vi "mainGUI.vi"() -> ()   [LabVIEW 2025]
uses:
  Photometrics/TPM-LabVIEWSamples/TPM LabVIEW adapter/Camera/Camera.lvclass
  Photometrics/TPM-LabVIEWSamples/TPM LabVIEW adapter/PVCAM/PVCAM.lvclass
  <userlib>/HOLOEYE SLM Display SDK 4.1.0/types/heds_slm_id_typedef.ctl
  <userlib>/HOLOEYE SLM Display SDK 4.1.0/types/heds_required_sdk_version_typedef.ctl
  <vilib>/Utility/error.llb/DialogType.ctl
  channel parameters cluster.ctl
  91398830-3a1b-4311-ae4e-d8b360d25ea5.vi
  <vilib>/DAQmx/write.llb/DAQmx Write (Analog DBL 1Chan 1Samp).vi
  <vilib>/DAQmx/write.llb/DAQmx Write (Analog Wfm 1Chan NSamp).vi
  <vilib>/DAQmx/write.llb/DAQmx Write (Analog 1D Wfm NChan NSamp).vi
  <vilib>/DAQmx/read.llb/DAQmx Read (Analog Wfm 1Chan NSamp).vi
  <vilib>/DAQmx/read.llb/DAQmx Read (Counter U32 1Chan 1Samp).vi
  <vilib>/DAQmx/write.llb/DAQmx Write (Analog 1D DBL NChan 1Samp).vi
  91398830-3a1b-4311-ae4e-d8b360d25ea5.vi/92577ae1-9a41-469a-bc80-42ec99e0da98.vi
  91398830-3a1b-4311-ae4e-d8b360d25ea5.vi/9add13f1-1b17-4127-a253-25fc8ec9b328.vi
  <userlib>/HOLOEYE SLM Display SDK 4.1.0/types/create_heds_data_flags_value.vi
  <userlib>/HOLOEYE SLM Display SDK 4.1.0/misc/heds_sdk_path_v4.1.vi
  <vilib>/Utility/Data Type/Get Type Information.vi
  <vilib>/Utility/Data Type/Get Cluster Information.vi
  <userlib>/HOLOEYE SLM Display SDK 4.1.0/misc/heds_check_error.vi
  <vilib>/DAQmx/miscellaneous.llb/DAQmx Fill In Error Info.vi
  <vilib>/DAQmx/create/channels.llb/DAQmx Create Channel (CI-Count Edges).vi
  <vilib>/DAQmx/create/channels.llb/DAQmx Create Channel (AO-Voltage-Basic).vi
  <vilib>/DAQmx/configure/trigger.llb/DAQmx Start Trigger (Digital Edge).vi
  <resource>/objmgr/daqmx.rc
  <vilib>/Analysis/NI_AALPro.lvlib
  <vilib>/vision/NI_Vision_Development_Module.lvlib
panel:
  in  "Dichroic/dual imaging":bool
  out "SLM image":picture
  out "Kinetix image":picture
  out "594 changed":bool=TRUE
  out "488 changed":bool=TRUE
  out "SLM ID":T1
  in  "Connect SLM":bool
  out "SLM connected":bool
  in  "488 nm LED control":dbl(slide) step=1.0 scale=0.0..100.0 scale format="%#_3g"
  out "Zelux image":picture
  in  "slow camera frequency":u16(ring)=10 caption="Hz" items=["10"=10, "20"=20, "50"=50]
  in  "File prefix":string
  out "488  nm voltage":dbl
  out "594 nm voltage":dbl
  in  "Connect Zelux":bool caption="Connect Kinetix"
  in  "Pulse Duty Cycle":dbl=50.0 caption="%" min=0.0 max=100.0 step=0.1
  in  "Pulse 488":bool
  in  "594 nm laser control":dbl(slide) step=1.0 scale=0.0..100.0 scale format="%#_3g"
  out "PVCam error out":errorcluster
  out "PVCAM Out":refnum<class "PVCAM.lvclass">
  out "Camera obj":refnum<class "Camera.lvclass">
  in  "Connect Kinetix":bool
  in  "Run time":i32 caption="s" min=0
  in  "Begin Experiment":bool
  in  "SLM high":bool
  in  "Load SLM image":bool
  in  "Create SLM image":bool
  in  "Save directory":path=path "D:/KinetixTest/SS_test"
  in  "# Trials":u32=1 caption="trials" min=1 step=1
  in  "Trial Time":dbl=0.1 caption="s" min=0.1 max=60.0 format="%#_2g"
  in  "Run Live":bool caption="Run live"
  in  "scan/fast camera frequency":u16(ring)=100 caption="Hz" items=["20"=20, "100"=100, "800"=800]
  in  "Galvo voltage":dbl=1.0 caption="V" min=0.1 max=1.8 format="%#_2g"
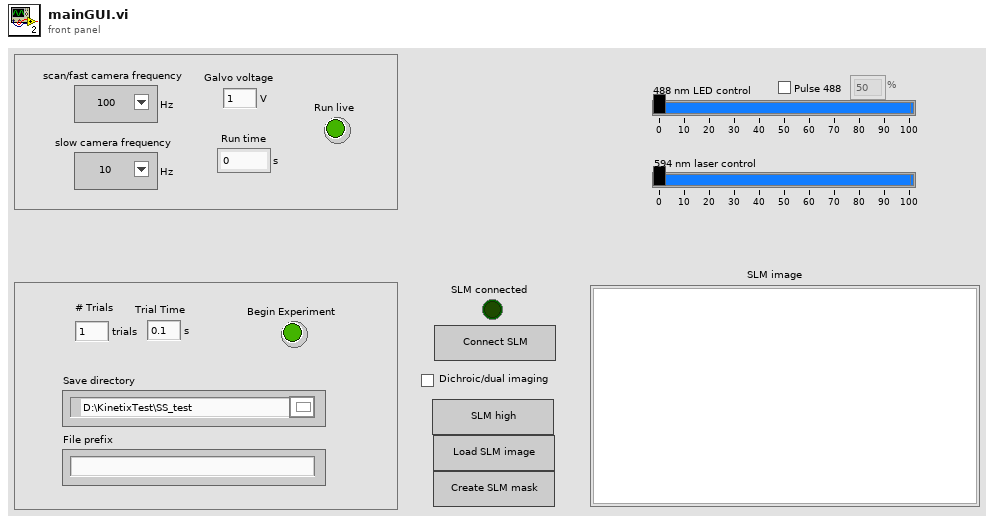
[diagram p1: front panel]
types:
  T1 = typedef "heds_slm_id_typedef.ctl" = cluster{"slmwindow_id":u32, "slmscreen_id":u32}
  T2 = typedef "IMAQ Image.ctl" = refnum<image>
  T3 = typedef "Image Type" = u32
  T4 = typedef "imagedata.ctl" = cluster{"image type":i32, "image depth":i32, "image":u8[], "mask":u8[], "colors":u32[], "Rectangle":cluster{"left":i16, "top":i16, "right":i16, "bottom":i16}}
  T5 = typedef "heds_required_sdk_version_typedef.ctl" = cluster{"Major Version Number":i32, "Minor Version Number":i32}
  T6 = enum8{"Enabled", "Disabled", "Disabled and Grayed Out"}
  T7 = enum16{"open", "open or create", "create or replace", "create", "open (read-only)"}
  T8 = typedef "DialogType.ctl" = u16
  T9 = cluster{"shutter trigger":refnum<k21>, "galvo control":refnum<k21>, "Kinetix trigger":refnum<k21>, "Kinetix readout":refnum<k21>, "Zelux trigger":refnum<k21>, "Zelux readout":refnum<k21>}
  T10 = typedef "channel parameters cluster.ctl" = cluster{"voltage":dbl, "frequency":dbl, "duty cycle":dbl, "sample rate":dbl}
  T11 = cluster{"maximum value":dbl, "minimum value":dbl}
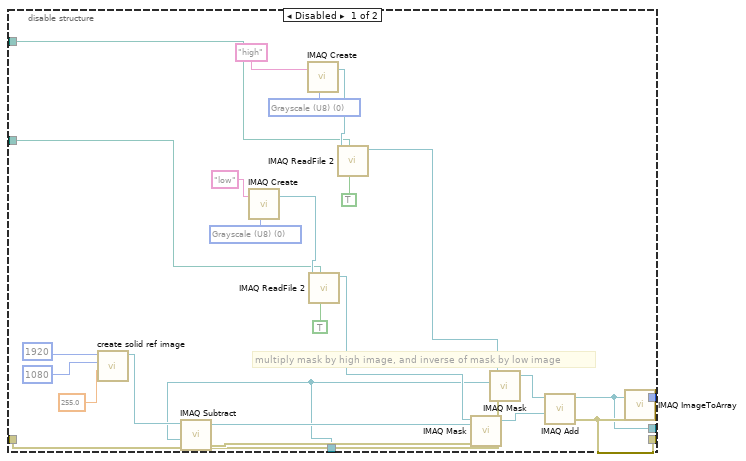
[diagram p3: hidden frame]
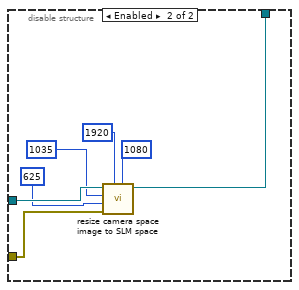
[diagram p4: hidden frame]
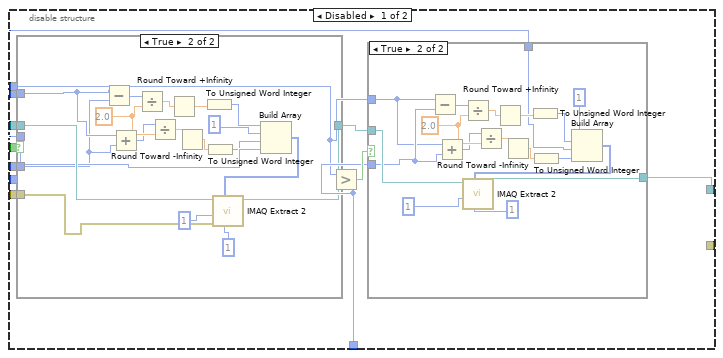
[diagram p5: hidden frame]
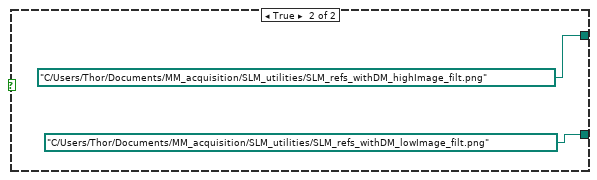
[diagram p8: hidden frame]
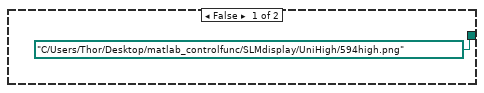
[diagram p10: hidden frame]
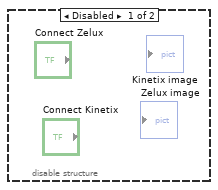
[diagram p14: hidden frame]
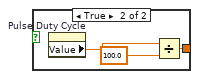
[diagram p17: hidden frame]
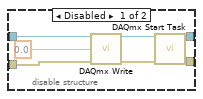
[diagram p18: hidden frame]
diagram:
  # "camera\nopen each in a different window? \n- shows live image\n- allows color scaling\n- allows application of ROI (default and custom)\n\n\n- during run, saves each frame"
  # "todo: \n\n** must stretch masks to fit SLM image\n- resize image based on SLM to camera conversion\n- add zero border to ROI mask if it is too small (assume correct center)\n- crop image if too large (assume correct center)\n\nMake main window not freeze after using slider\n\nstart ThorCam\n\nuse Kinetix without crashing program\n\ndisplay Kinetix and Thorcam during live\n\nin experiment, display and acquire both cameras \n- Kinetix by trial\n-Thorcam throughout\n\n\n\ncheck triggering from BPod (vs function generator - may need to change detection width etc)\n\n\nerror--checking\n- do not fail experiment if 1 camera fails \n\nnon-urgent: \nmake more elegant solution to finish final trial (currently using elapsed time)\nlog BPod trigger in (this is contained in Kinetix data, but can be separated for redundancy)\nadd timeouts for triggers\n\nsave metadata about experiment\n- start time\n- laser and LED power, pulse settings\n- SLM file used (if targeted)\n\nmake parameters file for hardcoded values\n \n\nsave timed experiment and metadata?"
  # "* should calibrate SLM *"
  n1 = case shown="True" "Create SLM image" {
    frame False {
    }
    frame True {
      n2 = flat-sequence {
        tunnel: [w39] -> w35
        tunnel: [w40] -> w34
        tunnel: [w59] -> w38
        tunnel: [w53] -> w37
        tunnel: [w52] -> w36
        tunnel: w35 -> [w46]
        tunnel: w34 -> [w49]
        tunnel: w38 -> [w197]
        tunnel: w37 -> [w196]
        tunnel: w36 -> [w195]
        frame #0 {
          n3 = local read "Save directory"() -> (w43:path)
          n4 = call "IMAQ Load Image Dialog"("Pattern"="*.tif*" ("pattern (all files)"), "Multiple Files? (No)"=FALSE, "Start Path"=w43) -> ("Path"=w42:path)  [unwired: 6 in, 2 out]
          n5 = call "create ROIs GUI.vi"("Mask high value (default 255)"=sgl 255.0, "TIFF path"=w42) -> ("error out"=w40:errorcluster, "ROI mask image"=w39:T2)  [unwired: 8 in]
        }
        frame #1 {
          w51 = 1035 ("y")
          # "if image is correct size or smaller: keep size\nassume center is the same\n\nif image is too large\n\nfinally, resize from image space to SLM space before multiplying with SLM reference images"
          n6 = local read "Dichroic/dual imaging"() -> (w62:bool)
          n7 = case shown="False" w62 {
            tunnel: [path "C:/Users/Thor/Desktop/matlab_controlfunc/SLMdisplay/UniHigh/594high.png" ("path to PNG file") path "C:/Users/Thor/Documents/MM_acquisition/SLM_utilities/SLM_refs_withDM_highImage_filt.png" ("path to PNG file")] -> w61
            tunnel: [path "C:/Users/Thor/Desktop/matlab_controlfunc/SLMdisplay/UniLow/594low.png" ("path to PNG file") path "C:/Users/Thor/Documents/MM_acquisition/SLM_utilities/SLM_refs_withDM_lowImage_filt.png" ("path to PNG file")] -> w60
            frame False {
            }
            frame True {
            }
          }
          n8 = call "IMAQ GetImageInfo"("Image"=w46) -> ("error out"=w57:errorcluster, "Y Resolution"=w54:i32, "X Resolution"=w56:i32)  [unwired: 3 in, 5 out]
          n9 = Greater?(x=w56, y=w51) -> (0:w58:bool)
          n10 = disable-structure shown="Enabled" {
            disable-tunnel: w58 -> [w133 _]
            disable-tunnel: w46 -> [w131 w178]
            disable-tunnel: w57 -> [w129 w175]
            disable-tunnel: w51 -> [w128 _]
            disable-tunnel: w56 -> [w127 w177]
            disable-tunnel: 625 ("y") -> [w126 w180]
            disable-tunnel: w54 -> [w125 w176]
            disable-tunnel: [w124 w173] -> w47
            disable-tunnel: w51 -> [_ w179]
            disable-tunnel: [_ w174] -> w50
            frame Disabled {
              n11 = case shown="True" w133 {
                tunnel: w131 -> [w153 w172]
                tunnel: [w153 w168] -> w130
                tunnel: w129 -> [_ w169]
                tunnel: w127 -> [_ w155]
                tunnel: w128 -> [_ w154]
                tunnel: w125 -> [_ w161]
                frame False {
                }
                frame True {
                  w160 = 2.0 ("y")
                  n12 = Subtract(x=w155, y=w154) -> (x-y=w166:i32)
                  n13 = Add(x=w155, y=w154) -> (x+y=w159:i32)
                  n14 = Divide(x=w166, y=w160) -> (x/y=w165:dbl)
                  n15 = Divide(x=w159, y=w160) -> (x/y=w158:dbl)
                  n16 = Round Toward +Infinity(x=w165) -> (ceil(x): smallest int >= x=w163:dbl)
                  n17 = Round Toward -Infinity(1:w158) -> (0:w157:dbl)
                  n18 = To Unsigned Word Integer(number=w163) -> (unsigned 16bit integer=w164:u16)
                  n19 = To Unsigned Word Integer(number=w157) -> (unsigned 16bit integer=w156:u16)
                  n20 = Build Array(w164, u16 1 ("element"), w156, w161) -> (w167:i32[])
                  n21 = call "IMAQ Extract 2"("Y Step Size"=1, "Optional Rectangle"=w167, "error in (no error)"=w169, "X Step Size"=1, "Image Src"=w172) -> ("Image Dst Out"=w168:T2)  [unwired: 5 in, 1 out]
                }
              }
              n22 = Greater?(x=w125, y=w126) -> (0:w132:bool)
              n23 = case shown="True" w132 {
                tunnel: w130 -> [w134 w152]
                tunnel: [w134 w151] -> w124
                tunnel: w127 -> [_ w138]
                tunnel: w126 -> [_ w137]
                tunnel: w125 -> [_ w136]
                frame False {
                }
                frame True {
                  w145 = 2.0 ("y")
                  n24 = Subtract(x=w136, y=w137) -> (x-y=w148:i32)
                  n25 = Add(x=w136, y=w137) -> (x+y=w144:i32)
                  n26 = Divide(x=w148, y=w145) -> (x/y=w147:dbl)
                  n27 = Divide(x=w144, y=w145) -> (x/y=w143:dbl)
                  n28 = Round Toward +Infinity(x=w147) -> (ceil(x): smallest int >= x=w146:dbl)
                  n29 = Round Toward -Infinity(1:w143) -> (0:w142:dbl)
                  n30 = To Unsigned Word Integer(number=w146) -> (unsigned 16bit integer=w141:u16)
                  n31 = To Unsigned Word Integer(number=w142) -> (unsigned 16bit integer=w140:u16)
                  n32 = Build Array(u16 1 ("element"), w141, w138, w140) -> (w135:i32[])
                  n33 = call "IMAQ Extract 2"("Y Step Size"=1, "Optional Rectangle"=w135, "X Step Size"=1, "Image Src"=w152) -> ("Image Dst Out"=w151:T2)  [unwired: 6 in, 1 out]
                }
              }
            }
            frame Enabled {
              n34 = call "crop_image_to_SLM_size.vi"("Y max"=w180, "X max"=w179, "error in (no error)"=w175, "Y size"=w176, "X size"=w177, "Image Src"=w178) -> ("error out"=w174:errorcluster, "Image Dst Out"=w173:T2)  [unwired: 4 in]
            }
          }
          n35 = disable-structure shown="Disabled" {
            disable-tunnel: w47 -> [w114 w123]
            disable-tunnel: [w99 w121] -> w48
            disable-tunnel: w50 -> [w93 w122]
            frame Disabled {
              w103 = 625 ("Y Resolution")
              w112 = 1035 ("X Resolution")
              n36 = call "IMAQ Create"("Image Name"="correctly sized image") -> ("New Image"=w116:T2)  [unwired: 4 in, 1 out]
              n37 = call "IMAQ GetImageInfo"("error in (no error)"=w93, "Image"=w114) -> ("Y Resolution"=w104:i32, "X Resolution"=w113:i32)  [unwired: 2 in, 6 out]
              n38 = Subtract(x=w112, y=w113) -> (x-y=w111:i32)
              n39 = call "IMAQ SetImageSize"("Y Resolution"=w103, "X Resolution"=w112, "Image"=w116) -> ("Image Out"=w115:T2)  [unwired: 2 in, 1 out]
              n40 = Subtract(x=w103, y=w104) -> (x-y=w108:i32)
              n41 = Divide(x=w111, y=2) -> (x/y=w109:dbl)
              n42 = Divide(x=w108, y=2) -> (x/y=w106:dbl)
              n43 = Round Toward -Infinity(1:w109) -> (0:w105:dbl)
              n44 = Round Toward -Infinity(1:w106) -> (0:w102:dbl)
              n45 = To Unsigned Word Integer(number=w105) -> (unsigned 16bit integer=w97:u16)
              n46 = To Unsigned Word Integer(number=w102) -> (unsigned 16bit integer=w96:u16)
              n47 = Build Array(w97, w96) -> (w95:u16[])
              n48 = call "IMAQ ImageToImage 2"("Offset Left/Top"=w95, "Image Src (Small)"=w114, "Image Src (Large)"=w115) -> ("Image Dst Out"=w98:T2)  [unwired: 7 in, 1 out]
              n49 = call "IMAQ Resample"("X Resolution"=1920, "Y Resolution"=1080, "Image Src"=w98) -> ("Image Dst Out"=w99:T2)  [unwired: 7 in, 1 out]
            }
            frame Enabled {
              n50 = call "resize camera space image to SLM space.vi"("Y SLM"=1080, "X SLM"=1920, "error in (no error)"=w122, "Y camera"=625, "X camera"=1035, "original image"=w123) -> ("Resized image"=w121:T2)  [unwired: 4 in, 1 out]
            }
          }
          n51 = disable-structure shown="Enabled" {
            disable-tunnel: w61 -> [w84 w92]
            disable-tunnel: w60 -> [w78 w91]
            disable-tunnel: [w74 w90] -> w59
            disable-tunnel: [w70 _] -> w53
            disable-tunnel: [w69 w89] -> w52
            disable-tunnel: w49 -> [w68 _]
            disable-tunnel: w48 -> [w63 w88]
            frame Disabled {
              w82 = T3 0 items=["Grayscale (U8)", "Grayscale (I16)", "Grayscale (SGL)", "Complex (CSG)", "RGB (U32)", "HSL (U32)", "RGB (U64)", "Grayscale (U16)"] ("Image Type")
              w87 = T3 0 items=["Grayscale (U8)", "Grayscale (I16)", "Grayscale (SGL)", "Complex (CSG)", "RGB (U32)", "HSL (U32)", "RGB (U64)", "Grayscale (U16)"] ("Image Type")
              # "multiply mask by high image, and inverse of mask by low image"
              n52 = call "create solid ref image.vi"("Pixel Value (default 255)"=sgl 255.0, "Y resolution"=1080 ("Y Resolution"), "X resolution"=1920 ("X Resolution")) -> ("solid image"=w67:T2)  [unwired: 7 in, 1 out]
              n53 = call "IMAQ Subtract"("Image Src A"=w67, "Image Src B"=w63, "error in (no error)"=w68) -> ("Image Dst Out"=w72:T2, "error out"=w75:errorcluster)  [unwired: 4 in]
              n54 = call "IMAQ Create"("Image Name"="low", "Image Type"=w82) -> ("New Image"=w81:T2)  [unwired: 3 in, 1 out]
              n55 = call "IMAQ Create"("Image Name"="high", "Image Type"=w87) -> ("New Image"=w86:T2)  [unwired: 3 in, 1 out]
              n56 = call "IMAQ ReadFile 2"("Use File Path Image Type"=TRUE, "File Path"=w78, "Image"=w81) -> ("Image Out"=w77:T2)  [unwired: 4 in, 4 out]
              n57 = call "IMAQ ReadFile 2"("Use File Path Image Type"=TRUE, "File Path"=w84, "Image"=w86) -> ("Image Out"=w76:T2)  [unwired: 4 in, 4 out]
              n58 = call "IMAQ Mask"("error in (no error)"=w75, "Image Mask"=w72, "Image Src"=w77) -> ("Image Dst Out"=w73:T2)  [unwired: 2 in, 1 out]
              n59 = call "IMAQ Mask"("error in (no error)"=w68, "Image Mask"=w63, "Image Src"=w76) -> ("Image Dst Out"=w71:T2)  [unwired: 2 in, 1 out]
              n60 = call "IMAQ Add"("Image Src A"=w71, "Image Src B"=w73) -> ("Image Dst Out"=w69:T2, "error out"=w70:errorcluster)  [unwired: 5 in]
              n61 = call "IMAQ ImageToArray"("error in (no error)"=w70, "Image"=w69) -> ("Image Pixels (U8)"=w74:u8[][])  [unwired: 2 in, 4 out]
            }
            frame Enabled {
              n62 = call "create SLM image from mask.vi"("low image path"=w91, "high image path"=w92, "Mask"=w88) -> ("Image Pixels (U8)"=w90:u8[][], "Final image"=w89:T2)  [unwired: 7 in]
            }
          }
        }
        frame #2 {
          n63 = property on="File prefix" class="Str"() -> ("Value"=w188:string)  [unwired: 2 in, 2 out]
          n64 = Format Date/Time String(time format string (%c)="%Y%m%d_%H%M%S.png") -> (date/time string=w187:string)  [unwired: 2 in]
          n65 = local read "SLM ID"() -> (w200:T1)
          n66 = Concatenate Strings("SLM_pattern_" ("string"), w188, w187) -> (w190:string)
          n67 = call "load_and_display_SLM.vi"("Image Data"=w197, "SLM ID"=w200) -> ("error out"=w198:errorcluster, "2D Picture"=w199:picture)  [unwired: 8 in]
          n68 = String To Path(string=w190) -> (path=w191:path)
          n69 = property on="Save directory" class="Path"() -> ("Value"=w193:path)  [unwired: 2 in, 2 out]
          n70 = Build Path(base path=w193, name or relative path=w191) -> (appended path=w192:path)
          n71 = property on="SLM image" class="Pict"(error in=w198, "Value"=w199) -> ()  [unwired: 1 in, 2 out]
          n72 = call-poly "IMAQ Write File 2"("Use bit depth? (false)"=TRUE, "error in (no error)"=w196, "Image Quality"=u32 1000, "File Path"=w192, "Image"=w195) -> ()  [unwired: 5 in, 2 out]
        }
        frame #3 {
          n73 = call "IMAQ Dispose"("All Images? (No)"=TRUE) -> ()  [unwired: 5 in, 1 out]
        }
      }
    }
  }
  n74 = case shown="True" "SLM high" {
    tunnel: "Dichroic/dual imaging" -> [_ w204]
    frame False {
    }
    frame True {
      n75 = case shown="True" w204 {
        tunnel: [path "C:/Users/Thor/Desktop/matlab_controlfunc/SLMdisplay/UniHigh/594high.png" ("path to PNG file") path "C:/Users/Thor/Documents/MM_acquisition/SLM_utilities/SLM_refs_withDM_highImage_filt.png" ("path to PNG file")] -> w203
        frame False {
        }
        frame True {
        }
      }
      n76 = call <vilib>:"Check if File or Folder Exists.vi"("path"=w203) -> ("file or folder exists?"=w202:bool)  [unwired: 8 in, 2 out]
      n77 = case shown="True" w202 {
        tunnel: w203 -> [_ w210]
        frame False {
        }
        frame True {
          n78 = call "png_file_to_image_array.vi"("dimension size 2"=1920 ("dimension size"), "dimension size 1"=1080 ("dimension size"), "path to PNG file"=w210) -> ("output array"=w207:u8[][])  [unwired: 8 in]
          n79 = local read "SLM ID"() -> (w213:T1)
          n80 = call "load_and_display_SLM.vi"("Image Data"=w207, "SLM ID"=w213) -> ("error out"=w211:errorcluster, "2D Picture"=w212:picture)  [unwired: 8 in]
          n81 = property on="SLM image" class="Pict"(error in=w211, "Value"=w212) -> ()  [unwired: 1 in, 2 out]
        }
      }
    }
  }
  n82 = case shown="True" "Load SLM image" {
    frame False {
    }
    frame True {
      n83 = property on="Save directory" class="Path"() -> ("Value"=w218:path)  [unwired: 2 in, 2 out]
      n84 = call "File Dialog"("start path"=w218, "pattern (all files)"="*.png") -> ("selected path"=w216:path, "exists"=w214:bool, "error out"=w215:errorcluster)  [unwired: 10 in, 1 out]
      n85 = case shown="True" w214 {
        tunnel: w216 -> [_ w230]
        tunnel: w215 -> [_ w229]
        frame False {
        }
        frame True {
          n86 = local read "SLM ID"() -> (w221:T1)
          n87 = call <vilib>:"Read PNG File.vi"("error in (no error)"=w229, "path to PNG file"=w230) -> ("image data"=w228:T4)  [unwired: 7 in, 2 out]
          n88 = Unbundle By Name(w228) -> ("image"=w226:u8[])  [unwired: 5 out]
          n89 = Reshape Array(w226, 1080 ("dimension size"), 1920 ("dimension size")) -> (w222:u8[][])
          n90 = call "heds_slm_show_imagedata.vim"("Image Data"=w222, "SLM ID"=w221) -> ("error out"=w220:errorcluster, "SLM ID out"=w219:T1)  [unwired: 7 in, 1 out]
          n91 = Unbundle By Name(w219) -> ("slmwindow_id"=w223:u32)
          n92 = call <userlib>:"heds_slmwindow_get_image_data.vi"("error in (no error)"=w220, "slmwindow_id"=w223) -> ("2D Picture"=→"SLM image":picture)  [unwired: 6 in, 3 out]
        }
      }
    }
  }
  n93 = case shown="True" "Connect SLM" {
    frame False {
    }
    frame True {
      n94 = call "connect_SLM.vi"("Required SDK version"=T5 {"Major Version Number"=4, "Minor Version Number"=1}) -> ("SLM connected"=w232:bool, "SLM ID"=→"SLM ID":T1)  [unwired: 9 in]
      "SLM connected" <- w232
      n95 = property on="SLM image" class="Pict"("ZoomFactor"=sgl 0.2 ("Zoom Factor")) -> ()  [unwired: 2 in, 2 out]
      n96 = case shown="True" w232 {
        frame False {
        }
        frame True {
          w235 = T6."Enabled" ("Disabled")
          n97 = property on="Create SLM image" class="Bool"("DisabledEnum"=w235) -> ()  [unwired: 2 in, 2 out]
          n98 = property on="SLM high" class="Bool"("DisabledEnum"=w235) -> ()  [unwired: 2 in, 2 out]
          n99 = property on="Load SLM image" class="Bool"("DisabledEnum"=w235) -> ()  [unwired: 2 in, 2 out]
        }
      }
    }
  }
  n100 = Divide(x="594 nm laser control", y=20.0) -> (x/y=→"594 nm voltage":dbl)
  n101 = disable-structure shown="Enabled" {
    frame Disabled {
    }
    frame Enabled {
    }
  }
  n102 = Divide(x="488 nm LED control", y=20.0) -> (x/y=→"488  nm voltage":dbl)
  n103 = Not(x="Pulse 488") -> (.not. x?=w18:bool)
  n104 = Boolean To (0,1)(Boolean=w18) -> (0, 1=w19:i16)
  n105 = Multiply(x=w19, y=2.0) -> (x*y=w20:dbl)
  n106 = property on="Pulse Duty Cycle" class="DigNum (strict)"("DisabledEnum"=w20) -> ()  [unwired: 2 in, 2 out]
  n107 = property on="Begin Experiment" class="Bool (strict)"() -> ("Value"=w10:bool)  [unwired: 2 in, 2 out]
  n108 = property on="Run Live" class="Bool (strict)"() -> ("Value"=w30:bool)  [unwired: 2 in, 2 out]
  n109 = Boolean To (0,1)(Boolean=w30) -> (0, 1=w31:i16)
  n110 = Boolean To (0,1)(Boolean=w10) -> (0, 1=w27:i16)
  n111 = case shown="True" w30 {
    tunnel: ["Run live" "End live"] -> w33
    frame False {
    }
    frame True {
    }
  }
  n112 = case shown="False" w10 {
    tunnel: ["Begin Experiment" "End experiment"] -> w25
    frame False {
    }
    frame True {
    }
  }
  n113 = Multiply(x=w31, y=2.0) -> (x*y=w29:dbl)
  n114 = Multiply(x=w27, y=2.0) -> (x*y=w26:dbl)
  n115 = property on="Begin Experiment" class="Bool (strict)"("DisabledEnum"=w29) -> ()  [unwired: 2 in, 2 out]
  n116 = property on="Run Live" class="Bool (strict)"("DisabledEnum"=w26) -> ()  [unwired: 2 in, 2 out]
  n117 = disable-structure shown="Enabled" {
    disable-tunnel: w10 -> [w245 _]
    disable-tunnel: "Trial Time" -> [w244 _]
    disable-tunnel: "scan/fast camera frequency" -> [w243 _]
    disable-tunnel: "slow camera frequency" -> [w242 _]
    disable-tunnel: "# Trials" -> [w241 _]
    disable-tunnel: "Galvo voltage" -> [w240 _]
    frame Disabled {
      n118 = case shown="True" w245 {
        tunnel: w243 -> [_ w414]
        tunnel: w240 -> [_ w413]
        tunnel: w244 -> [_ w272]
        tunnel: w241 -> [_ w412]
        tunnel: w242 -> [_ w291]
        tunnel: w242 -> [_ w269]
        frame False {
        }
        frame True {
          w307 = T8 0 items=["no dialog", "OK message", "continue or stop message", "OK message + warnings", "continue/stop + warnings"] ("type of dialog (OK msg:1)")
          w313 = 10123 items=["Finite Samples"=10178, "Continuous Samples"=10123, "Hardware Timed Single Point"=12522] ("SampQuant.SampMode")
          w318 = T8 0 items=["no dialog", "OK message", "continue or stop message", "OK message + warnings", "continue/stop + warnings"] ("type of dialog (OK msg:1)")
          w325 = 10123 items=["Finite Samples"=10178, "Continuous Samples"=10123, "Hardware Timed Single Point"=12522] ("SampQuant.SampMode")
          w337 = 10178 items=["Finite Samples"=10178, "Continuous Samples"=10123, "Hardware Timed Single Point"=12522] ("SampQuant.SampMode")
          w278 = 10178 items=["Finite Samples"=10178, "Continuous Samples"=10123, "Hardware Timed Single Point"=12522] ("SampQuant.SampMode")
          w350 = 10123 items=["Finite Samples"=10178, "Continuous Samples"=10123, "Hardware Timed Single Point"=12522] ("SampQuant.SampMode")
          w373 = 10280 items=["Rising"=10280, "Falling"=10171] ("edge")
          w261 = tag "/GalvoPMT/PFI9" ("source")
          w356 = 10178 items=["Finite Samples"=10178, "Continuous Samples"=10123, "Hardware Timed Single Point"=12522] ("SampQuant.SampMode")
          w408 = T8 0 items=["no dialog", "OK message", "continue or stop message", "OK message + warnings", "continue/stop + warnings"] ("type of dialog (OK msg:1)")
          w410 = T8 0 items=["no dialog", "OK message", "continue or stop message", "OK message + warnings", "continue/stop + warnings"] ("type of dialog (OK msg:1)")
          # "min pulse width ensures proper increment/debouncing"
          n119 = call-poly <vilib>:"DAQmx Create Virtual Channel.vi"("maximum value"=5.0, "minimum value"=0.0, "physical channels"=tag "PZT/ao0", "name to assign"="488 nm") -> ("task out"=w289:refnum<k21>, "error out"=w290:errorcluster)  [unwired: 10 in]
          n120 = property class="DAQmx Timing"(reference=w289, error in=w290, "Sample Quantity:Sample Mode"=w325) -> (reference out=w323:refnum<k21>, error out=w322:errorcluster)
          n121 = property on="488  nm voltage" class="DigNum (strict)"() -> ("Value"=w293:dbl)  [unwired: 2 in, 2 out]
          n122 = property on="Pulse 488" class="Bool (strict)"() -> ("Value"=w326:bool)  [unwired: 2 in, 2 out]
          n123 = case shown="True" w326 {
            tunnel: [w416 w425] -> w324
            tunnel: w323 -> [w418 w427]
            tunnel: [w415 w424] -> w321
            tunnel: w322 -> [w419 w428]
            tunnel: w293 -> [w417 w430]
            tunnel: w291 -> [_ w420]
            frame False {
              n124 = call-poly <vilib>:"DAQmx Write.vi"("task/channels in"=w418, "data"=w417, "error in"=w419) -> ("task out"=w416:refnum<k21>, "error out"=w415:errorcluster)  [unwired: 10 in, 1 out]
            }
            frame True {
              # "need to copy loop in free run case (after fixing it)"
              n125 = property on="Pulse Duty Cycle" class="DigNum (strict)"() -> ("Value"=w423:dbl)  [unwired: 2 in, 2 out]
              n126 = property class="DAQmx Timing"(reference=w427) -> ("SampClk.Rate"=w429:dbl)  [unwired: 1 in, 2 out]
              n127 = Divide(x=w423, y=100.0) -> (x/y=w421:dbl)
              n128 = Divide(x=1.0, y=w420) -> (x/y=w431:dbl)
              n129 = call "make step function for duty cycle.vi"("amplitude"=w430, "period"=w431, "duty cycle"=w421, "sample rate"=w429) -> ("Waveform out"=w426:waveform(dbl))  [unwired: 7 in]
              n130 = call-poly <vilib>:"DAQmx Write.vi"("task/channels in"=w427, "data"=w426, "error in"=w428) -> ("task out"=w425:refnum<k21>, "error out"=w424:errorcluster)  [unwired: 10 in, 1 out]
            }
          }
          n131 = call "init_DAQ_cluster.vi"("Sample rate"=100000.0, "Slow/Zelux frame frequency"=w269, "Fast/Kinetix frame frequency"=w414) -> ("error out"=w270:errorcluster, "tasks cluster"=w274:T9)  [unwired: 7 in]
          n132 = Unbundle By Name(w274) -> ("shutter trigger"=w273:refnum<k21>, "galvo control"=w254:refnum<k21>, "Kinetix trigger"=w256:refnum<k21>, "Zelux trigger"=w260:refnum<k21>, "Kinetix readout"=w257:refnum<k21>, "Zelux readout"=w258:refnum<k21>)
          n133 = property class="DAQmx Timing"(reference=w254) -> ("SampClk.Rate"=w338:dbl)  [unwired: 1 in, 2 out]
          n134 = call-poly <vilib>:"DAQmx Trigger.vi"("task/channels in"=w254, "source"=w261, "error in"=w270) -> ("task out"=w405:refnum<k21>, "error out"=w404:errorcluster)  [unwired: 11 in]
          n135 = property on="File prefix" class="Str"() -> ("Value"=w263:string)  [unwired: 2 in, 2 out]
          n136 = property class="DAQmx Channel"(reference=w260, error in=w270) -> ("CO.Pulse.Freq"=w271:dbl)  [unwired: 2 out]
          n137 = property class="DAQmx Channel"(reference=w256, error in=w270) -> ("CO.Pulse.Freq"=w292:dbl)  [unwired: 2 out]
          n138 = property class="DAQmx Timing"(reference=w254) -> ("SampClk.Rate"=w353:dbl)  [unwired: 1 in, 2 out]
          n139 = property class="DAQmx Trigger"(reference=w405, error in=w404, "Start.Retriggerable"=TRUE) -> (reference out=w361:refnum<k21>)  [unwired: 1 out]
          n140 = Concatenate Strings(w263, "_Kinetix.tdms") -> (w268:string)
          n141 = Concatenate Strings(w263, "_Zelux.tdms") -> (w264:string)
          n142 = call-poly <vilib>:"DAQmx Create Virtual Channel.vi"("maximum value"=5.0, "minimum value"=0.0, "physical channels"=tag "PZT/ao1", "name to assign"="594 nm") -> ("task out"=w315:refnum<k21>, "error out"=w314:errorcluster)  [unwired: 10 in]
          n143 = Divide(x=1.0, y=w272) -> (x/y=w370:dbl)
          n144 = Multiply(x=w271, y=w272) -> ()  [unwired: 1 out]
          n145 = property class="DAQmx Channel"(reference=w273, error in=w270, "CO.Pulse.Freq"=w370) -> (reference out=w372:refnum<k21>)  [unwired: 1 out]
          n146 = property on="594 nm voltage" class="DigNum (strict)"() -> ("Value"=w316:dbl)  [unwired: 2 in, 2 out]
          n147 = Multiply(x=w292, y=w272) -> (x*y=w354:dbl)
          n148 = Multiply(x=w353, y=w272) -> (x*y=w355:dbl)
          n149 = String To Path(string=w268) -> (path=w266:path)
          n150 = String To Path(string=w264) -> (path=w265:path)
          n151 = call-poly <vilib>:"DAQmx Trigger.vi"("task/channels in"=w256, "source"=w261) -> ("task out"=w391:refnum<k21>, "error out"=w390:errorcluster)  [unwired: 12 in]
          n152 = call "galvo_triangle_wave.vi"("trial seconds"=w272, "final frequency"=w292, "amplitude"=w413, "sample rate"=w353) -> ("waveform array out"=w367:waveform(dbl)[])  [unwired: 7 in]
          n153 = property class="DAQmx Trigger"(reference=w391, error in=w390, "Start.Retriggerable"=TRUE) -> (reference out=w357:refnum<k21>, error out=w358:errorcluster)
          n154 = call-poly <vilib>:"DAQmx Write.vi"("task/channels in"=w315, "data"=w316, "error in"=w314) -> ("task out"=w312:refnum<k21>, "error out"=w311:errorcluster)  [unwired: 10 in, 1 out]
          n155 = call-poly <vilib>:"DAQmx Create Virtual Channel.vi"("initial count"=u32 0, "edge"=w373, "counter"=tag "GalvoPMT/ctr1") -> ("task out"=w402:refnum<k21>, "error out"=w401:errorcluster)  [unwired: 11 in]
          n156 = call-poly <vilib>:"DAQmx Trigger.vi"("task/channels in"=w372, "source"=w261) -> ("task out"=w388:refnum<k21>, "error out"=w389:errorcluster)  [unwired: 12 in]
          n157 = property on="Save directory" class="Path"() -> ("Value"=w349:path)  [unwired: 2 in, 2 out]
          n158 = property on="Save directory" class="Path"() -> ("Value"=w284:path)  [unwired: 2 in, 2 out]
          n159 = property class="DAQmx Timing"(reference=w361, "Sample Quantity:Sample Mode"=w356, "SampQuant.SampPerChan"=w355) -> (reference out=w362:refnum<k21>)  [unwired: 1 in, 1 out]
          n160 = property class="DAQmx Channel"(reference=w402, error in=w401, "CI.CountEdges.Term"=w261, "CI.CountEdges.DigFltr.MinPulseWidth"=1e-06 ("DI.DigFltr.MinPulseWidth")) -> (reference out=w395:refnum<k21>, error out=w394:errorcluster)
          n161 = property class="DAQmx Trigger"(reference=w388, error in=w389, "Start.Retriggerable"=TRUE) -> (reference out=w387:refnum<k21>)  [unwired: 1 out]
          n162 = Build Path(base path=w349, name or relative path=w266) -> (appended path=w345:path)
          n163 = Build Path(base path=w284, name or relative path=w265) -> (appended path=w283:path)
          n164 = call-poly <vilib>:"DAQmx Trigger.vi"("task/channels in"=w257, "source"=w261) -> ("task out"=w248:refnum<k21>, "error out"=w346:errorcluster)  [unwired: 12 in]
          n165 = call-poly <vilib>:"DAQmx Trigger.vi"("task/channels in"=w258, "source"=w261) -> ("task out"=w251:refnum<k21>, "error out"=w250:errorcluster)  [unwired: 12 in]
          n166 = Multiply(x=w272, y=w338) -> (x*y=w277:dbl)
          n167 = property class="DAQmx Timing"(reference=w357, error in=w358, "Sample Quantity:Sample Mode"=w337, "SampQuant.SampPerChan"=w354) -> (reference out=w360:refnum<k21>, error out=w359:errorcluster)
          n168 = property class="DAQmx Timing"(reference=w248, "Sample Quantity:Sample Mode"=w278, "SampQuant.SampPerChan"=w277) -> (reference out=w247:refnum<k21>)  [unwired: 1 in, 1 out]
          n169 = property class="DAQmx Timing"(reference=w251, error in=w250, "Sample Quantity:Sample Mode"=w278, "SampQuant.SampPerChan"=w277) -> (reference out=w253:refnum<k21>, error out=w249:errorcluster)
          n170 = property class="DAQmx Timing"(reference=w312, error in=w311, "Sample Quantity:Sample Mode"=w313) -> (reference out=w310:refnum<k21>, error out=w309:errorcluster)
          n171 = call-poly <vilib>:"DAQmx Write.vi"("task/channels in"=w362, "data"=w367, "error in"=w270) -> ("task out"=w366:refnum<k21>, "error out"=w365:errorcluster)  [unwired: 10 in, 1 out]
          n172 = property class="DAQmx Trigger"(reference=w247, "Start.Retriggerable"=TRUE) -> (reference out=w259:refnum<k21>)  [unwired: 1 in, 1 out]
          n173 = property class="DAQmx Trigger"(reference=w253, error in=w249, "Start.Retriggerable"=TRUE) -> (reference out=w276:refnum<k21>, error out=w275:errorcluster)
          n174 = call <vilib>:"DAQmx Start Task.vi"("task/channels in"=w360, "error in"=w359) -> ("task out"=w382:refnum<k21>, "error out"=w381:errorcluster)  [unwired: 12 in]
          n175 = call <vilib>:"DAQmx Start Task.vi"("task/channels in"=w395, "error in"=w394) -> ("task out"=w393:refnum<k21>, "error out"=w392:errorcluster)  [unwired: 12 in]
          n176 = call <vilib>:"DAQmx Start Task.vi"("task/channels in"=w310, "error in"=w309) -> ("task out"=w305:refnum<k21>, "error out"=w304:errorcluster)  [unwired: 12 in]
          n177 = call <vilib>:"DAQmx Start Task.vi"("task/channels in"=w366, "error in"=w365) -> ("task out"=w364:refnum<k21>, "error out"=w363:errorcluster)  [unwired: 12 in]
          n178 = call <vilib>:"DAQmx Start Task.vi"("task/channels in"=w387, "error in"=w270) -> ("task out"=w378:refnum<k21>, "error out"=w375:errorcluster)  [unwired: 12 in]
          n179 = TDMS Open(10:T7."open or create" ("operation (0:open)"), 11:w345) -> (0:w342:errorcluster, 3:w344:refnum<k34>)  [unwired: 5 in]
          n180 = TDMS Open(10:T7."open or create" ("operation (0:open)"), 11:w283) -> (0:w279:errorcluster, 3:w282:refnum<k34>)  [unwired: 5 in]
          n181 = call <vilib>:"DAQmx Start Task.vi"("task/channels in"=w324, "error in"=w321) -> ("task out"=w320:refnum<k21>, "error out"=w317:errorcluster)  [unwired: 12 in]
          n182 = while {
            tunnel: w412 -> [w459]
            tunnel: [w483] -> w399
            tunnel: [w482] -> w397
            tunnel: w393 -> [w479]
            tunnel: w392 -> [w478]
            tunnel: [w472] -> w384
            tunnel: [w469] -> w383
            tunnel: w382 -> [w476]
            tunnel: w381 -> [w477]
            tunnel: [w477] -> w380
            tunnel: [w476] -> w379
            tunnel: w378 -> [w468]
            tunnel: [w468] -> w377
            tunnel: [w475] -> w376
            tunnel: w375 -> [w475]
            tunnel: [FALSE] -> w369
            tunnel: w364 -> [w469]
            tunnel: w363 -> [w472]
            tunnel: w272 -> [w467]
            tunnel: w259 -> [w461]
            tunnel: w344 -> [w465]
            tunnel: [w464] -> w343
            tunnel: w342 -> [w466]
            tunnel: [w463] -> w341
            tunnel: [w462] -> w340
            tunnel: w277 -> [_]
            tunnel: [w457] -> w297
            tunnel: w320 -> [w457]
            tunnel: [w456] -> w296
            tunnel: w317 -> [w456]
            tunnel: [w455] -> w306
            tunnel: w305 -> [w455]
            tunnel: w304 -> [w454]
            tunnel: [w454] -> w303
            tunnel: [w453] -> w288
            tunnel: [w452] -> w287
            tunnel: w282 -> [w451]
            tunnel: [w450] -> w280
            tunnel: w279 -> [w449]
            tunnel: w276 -> [w436]
            stop <- w474 stop-if-true
            # "Run experiment"
            n183 = call-poly <vilib>:"DAQmx Read.vi"("task/channels in"=w479, "error in"=w478) -> ("task out"=w483:refnum<k21>, "data"=w481:u32, "error out"=w482:errorcluster)  [unwired: 11 in]
            n184 = call-poly <vilib>:"DAQmx Read.vi"("task/channels in"=w461) -> ("task out"=w462:refnum<k21>, "data"=w434:waveform(dbl))  [unwired: 12 in, 1 out]
            n185 = call-poly <vilib>:"DAQmx Read.vi"("task/channels in"=w436) -> ("task out"=w450:refnum<k21>, "data"=w433:waveform(dbl))  [unwired: 12 in, 1 out]
            n186 = Subtract(x=w459, y=u32 1) -> (x-y=w458:u32)
            n187 = Wait (ms)(milliseconds to wait=u32 10) -> ()  [unwired: 1 out]
            n188 = Greater Or Equal?(x=w481, y=w458) -> (x >= y?=w471:bool)
            n189 = Unbundle By Name(w434) -> ("t0"=w443:timestamp, "dt"=w446:dbl)  [unwired: 1 out]
            n190 = Unbundle By Name(w433) -> ("t0"=w437:timestamp, "dt"=w440:dbl)  [unwired: 1 out]
            n191 = call <vilib>:"Threshold Detector.vi"("threshold"=1.0, "X"=w434) -> ("Indices"=w447:i32[])  [unwired: 1 in, 2 out]
            n192 = call <vilib>:"Threshold Detector.vi"("threshold"=1.0, "X"=w433) -> ("Indices"=w441:i32[])  [unwired: 1 in, 2 out]
            n193 = Multiply(x=w447, y=w446) -> (x*y=w445:dbl[])
            n194 = Multiply(x=w441, y=w440) -> (x*y=w439:dbl[])
            n195 = case shown="True" w471 {
              selector: w471 -> [w485 _]
              tunnel: [w485 w487] -> w470
              tunnel: w467 -> [_ w486]
              frame False {
              }
              frame True {
                n196 = while {
                  tunnel: [w488] -> w487
                  tunnel: w486 -> [w489]
                  stop <- w488 stop-if-true
                  n197 = call "Elapsed Time"("Time Target (s)"=w489) -> ("Time has Elapsed"=w488:bool)  [unwired: 11 in, 7 out]
                }
              }
            }
            n198 = Add(x=w445, y=w443) -> (x+y=w448:timestamp[])
            n199 = Add(x=w439, y=w437) -> (x+y=w442:timestamp[])
            n200 = TDMS Write(0:w465, 9:w448, 11:w466) -> (4:w464:refnum<k34>, 15:w463:errorcluster)  [unwired: 3 in, 2 out]
            n201 = TDMS Write(0:w451, 9:w442, 11:w449) -> (4:w452:refnum<k34>, 15:w453:errorcluster)  [unwired: 3 in, 2 out]
            n202 = property on="Begin Experiment" class="Bool (strict)"() -> ("Value"=w435:bool)  [unwired: 2 in, 2 out]
            n203 = Not(x=w435) -> (.not. x?=w484:bool)
            n204 = Or(x=w470, y=w484) -> (x .or. y?=w474:bool)
          }
          n205 = property on="Begin Experiment" class="Bool (strict)"("Value"=w369) -> ()  [unwired: 2 in, 2 out]
          n206 = TDMS Close(8:w341, 11:w343) -> ()  [unwired: 2 out]
          n207 = TDMS Close(8:w288, 11:w287) -> ()  [unwired: 2 out]
          n208 = call <vilib>:"DAQmx Stop Task.vi"("task/channels in"=w379, "error in"=w380) -> ("task out"=w406:refnum<k21>, "error out"=w407:errorcluster)  [unwired: 12 in]
          n209 = call <vilib>:"DAQmx Stop Task.vi"("task/channels in"=w399, "error in"=w397) -> ("task out"=w398:refnum<k21>, "error out"=w396:errorcluster)  [unwired: 12 in]
          n210 = call <vilib>:"DAQmx Stop Task.vi"("task/channels in"=w297, "error in"=w296) -> ("task out"=w300:refnum<k21>, "error out"=w301:errorcluster)  [unwired: 12 in]
          n211 = call <vilib>:"DAQmx Clear Task.vi"("task in"=w306, "error in"=w303) -> ("error out"=w308:errorcluster)  [unwired: 13 in]
          n212 = call <vilib>:"DAQmx Stop Task.vi"("task/channels in"=w383, "error in"=w384) -> ("task out"=w352:refnum<k21>, "error out"=w351:errorcluster)  [unwired: 12 in]
          n213 = call <vilib>:"DAQmx Clear Task.vi"("task in"=w377, "error in"=w376) -> ("error out"=w409:errorcluster)  [unwired: 13 in]
          n214 = call <vilib>:"DAQmx Stop Task.vi"("task/channels in"=w340, "error in"=w346) -> ("task out"=w348:refnum<k21>, "error out"=w347:errorcluster)  [unwired: 12 in]
          n215 = call <vilib>:"DAQmx Stop Task.vi"("task/channels in"=w280, "error in"=w275) -> ("task out"=w286:refnum<k21>, "error out"=w285:errorcluster)  [unwired: 12 in]
          n216 = call <vilib>:"DAQmx Clear Task.vi"("task in"=w398, "error in"=w396) -> ()  [unwired: 13 in, 1 out]
          n217 = call <vilib>:"DAQmx Clear Task.vi"("task in"=w348, "error in"=w347) -> ()  [unwired: 13 in, 1 out]
          n218 = call <vilib>:"DAQmx Clear Task.vi"("task in"=w286, "error in"=w285) -> ()  [unwired: 13 in, 1 out]
          n219 = call <vilib>:"DAQmx Clear Task.vi"("task in"=w406, "error in"=w407) -> ("error out"=w411:errorcluster)  [unwired: 13 in]
          n220 = call <vilib>:"Simple Error Handler.vi"("type of dialog (OK msg:1)"=w307, "error in (no error)"=w308) -> ()  [unwired: 3 in, 5 out]
          n221 = property class="DAQmx Timing"(reference=w352, error in=w351, "Sample Quantity:Sample Mode"=w350) -> (reference out=w336:refnum<k21>, error out=w335:errorcluster)
          n222 = call <vilib>:"Simple Error Handler.vi"("type of dialog (OK msg:1)"=w408, "error in (no error)"=w409) -> ()  [unwired: 3 in, 5 out]
          n223 = call-poly <vilib>:"DAQmx Write.vi"("task/channels in"=w300, "data"=0.0, "error in"=w301) -> ("task out"=w299:refnum<k21>, "error out"=w298:errorcluster)  [unwired: 10 in, 1 out]
          n224 = call <vilib>:"Simple Error Handler.vi"("type of dialog (OK msg:1)"=w410, "error in (no error)"=w411) -> ()  [unwired: 3 in, 5 out]
          n225 = call <vilib>:"DAQmx Start Task.vi"("task/channels in"=w299, "error in"=w298) -> ("task out"=w295:refnum<k21>, "error out"=w294:errorcluster)  [unwired: 12 in]
          n226 = call "galvo_recenter.vi"("error in"=w335, "task/channels in"=w336) -> ()  [unwired: 10 in]
          n227 = call <vilib>:"DAQmx Clear Task.vi"("task in"=w295, "error in"=w294) -> ("error out"=w319:errorcluster)  [unwired: 13 in]
          n228 = call <vilib>:"Simple Error Handler.vi"("type of dialog (OK msg:1)"=w318, "error in (no error)"=w319) -> ()  [unwired: 3 in, 5 out]
        }
      }
    }
    frame Enabled {
    }
  }
  n229 = disable-structure shown="Enabled" {
    disable-tunnel: w10 -> [w495 _]
    disable-tunnel: "Trial Time" -> [w494 _]
    disable-tunnel: "# Trials" -> [w493 _]
    disable-tunnel: "Galvo voltage" -> [w492 _]
    disable-tunnel: "slow camera frequency" -> [w491 _]
    disable-tunnel: "scan/fast camera frequency" -> [w490 _]
    frame Enabled {
      n230 = case shown="True" w495 {
        tunnel: w490 -> [_ w685]
        tunnel: w492 -> [_ w565]
        tunnel: w494 -> [_ w561]
        tunnel: w493 -> [_ w611]
        tunnel: w491 -> [_ w614]
        frame False {
        }
        frame True {
          w538 = 10123 items=["Finite Samples"=10178, "Continuous Samples"=10123, "Hardware Timed Single Point"=12522] ("SampQuant.SampMode")
          w546 = 10150 items=["Analog Edge"=10099, "Analog Multi Edge"=16108, "Digital Edge"=10150, "Digital Pattern"=10398, "Analog Window"=10103, "Time"=15996, "None"=10230] ("Start.TrigType")
          w557 = 10388 items=["Sample Clock"=10388, "Burst Handshake"=12548, "Handshake"=10389, "Implicit"=10451, "On Demand"=10390, "Change Detection"=12504, "Pipelined Sample Clock"=14668] ("SampTimingType")
          w580 = T8 0 items=["no dialog", "OK message", "continue or stop message", "OK message + warnings", "continue/stop + warnings"] ("type of dialog (OK msg:1)")
          w589 = T8 0 items=["no dialog", "OK message", "continue or stop message", "OK message + warnings", "continue/stop + warnings"] ("type of dialog (OK msg:1)")
          w625 = T8 0 items=["no dialog", "OK message", "continue or stop message", "OK message + warnings", "continue/stop + warnings"] ("type of dialog (OK msg:1)")
          w642 = 10123 items=["Finite Samples"=10178, "Continuous Samples"=10123, "Hardware Timed Single Point"=12522] ("SampQuant.SampMode")
          w645 = T8 0 items=["no dialog", "OK message", "continue or stop message", "OK message + warnings", "continue/stop + warnings"] ("type of dialog (OK msg:1)")
          w648 = 10178 items=["Finite Samples"=10178, "Continuous Samples"=10123, "Hardware Timed Single Point"=12522] ("SampQuant.SampMode")
          w671 = 10280 items=["Rising"=10280, "Falling"=10171] ("edge")
          w604 = TRUE ("Start.Retriggerable")
          w528 = tag "/GalvoPMT/PFI9" ("source")
          w508 = 10178 items=["Finite Samples"=10178, "Continuous Samples"=10123, "Hardware Timed Single Point"=12522] ("SampQuant.SampMode")
          # "need to copy loop in free run case (after fixing it)"
          # "stop trial count"
          # "stop 488 LED"
          # "stop 594 laser"
          # "stop Zelux trigger"
          # "stop Kinetix trigger"
          # "close shutter"
          # "stop and park galvos"
          # "close Kinetix logging file"
          # "close Zelux logging file"
          # "min pulse width ensures proper increment/debouncing"
          n231 = call "init_DAQ_cluster.vi"("Sample rate"=100000.0, "Slow/Zelux frame frequency"=w614, "Fast/Kinetix frame frequency"=w685) -> ("error out"=w527:errorcluster, "tasks cluster"=w627:T9)  [unwired: 7 in]
          n232 = Divide(x=1.0, y=w561) -> (x/y=w669:dbl)
          n233 = call-poly <vilib>:"DAQmx Create Virtual Channel.vi"("maximum value"=5.0, "minimum value"=0.0, "physical channels"=tag "PZT/ao0", "name to assign"="488 nm") -> ("task out"=w553:refnum<k21>, "error out"=w552:errorcluster)  [unwired: 10 in]
          n234 = property class="DAQmx Timing"(reference=w553) -> ("SampClk.Rate"=w558:dbl)  [unwired: 1 in, 2 out]
          n235 = Unbundle By Name(w627) -> ("shutter trigger"=w613:refnum<k21>, "galvo control"=w567:refnum<k21>, "Kinetix trigger"=w568:refnum<k21>, "Zelux trigger"=w569:refnum<k21>, "Kinetix readout"=w610:refnum<k21>, "Zelux readout"=w595:refnum<k21>)
          n236 = property class="DAQmx Channel"(reference=w569) -> ("CO.Pulse.Freq"=w594:dbl)  [unwired: 1 in, 2 out]
          n237 = property class="DAQmx Channel"(reference=w568) -> ("CO.Pulse.Freq"=w596:dbl)  [unwired: 1 in, 2 out]
          n238 = Multiply(x=w558, y=w561) -> (x*y=w562:dbl)
          n239 = property class="DAQmx Channel"(reference=w613, "CO.Pulse.Freq"=w669) -> (reference out=w612:refnum<k21>)  [unwired: 1 in, 1 out]
          n240 = property class="DAQmx Timing"(reference=w553, error in=w552, "Sample Quantity:Sample Mode"=w648, "SampQuant.SampPerChan"=w562, "SampClk.Src"=tag "OnboardClock", "SampClk.Rate"=w558, "SampTimingType"=w557) -> (reference out=w548:refnum<k21>, error out=w547:errorcluster)
          n241 = Multiply(x=w596, y=w561) -> (x*y=w592:dbl)
          n242 = Multiply(x=w594, y=w561) -> (x*y=w593:dbl)
          n243 = property class="DAQmx Trigger"(reference=w548, error in=w547, "Start.Retriggerable"=TRUE, "Start.TrigType"=w546) -> (reference out=w549:refnum<k21>, error out=w550:errorcluster)
          n244 = call-poly <vilib>:"DAQmx Trigger.vi"("task/channels in"=w612, "source"=w528, "error in"=w527) -> ("task out"=w675:refnum<k21>, "error out"=w526:errorcluster)  [unwired: 11 in]
          n245 = call-poly <vilib>:"DAQmx Trigger.vi"("task/channels in"=w569, "source"=w528, "error in"=w527) -> ("task out"=w607:refnum<k21>, "error out"=w523:errorcluster)  [unwired: 11 in]
          n246 = call-poly <vilib>:"DAQmx Trigger.vi"("task/channels in"=w568, "source"=w528, "error in"=w527) -> ("task out"=w608:refnum<k21>, "error out"=w524:errorcluster)  [unwired: 11 in]
          n247 = call-poly <vilib>:"DAQmx Trigger.vi"("task/channels in"=w610, "source"=w528, "error in"=w527) -> ("task out"=w606:refnum<k21>, "error out"=w522:errorcluster)  [unwired: 11 in]
          n248 = call-poly <vilib>:"DAQmx Trigger.vi"("task/channels in"=w567, "source"=w528, "error in"=w527) -> ("task out"=w684:refnum<k21>, "error out"=w525:errorcluster)  [unwired: 11 in]
          n249 = call-poly <vilib>:"DAQmx Trigger.vi"("task/channels in"=w595, "source"=w528, "error in"=w527) -> ("task out"=w605:refnum<k21>, "error out"=w521:errorcluster)  [unwired: 11 in]
          n250 = property on="Pulse 488" class="Bool (strict)"() -> ("Value"=w533:bool)  [unwired: 2 in, 2 out]
          n251 = call-poly <vilib>:"DAQmx Create Virtual Channel.vi"("maximum value"=5.0, "minimum value"=0.0, "physical channels"=tag "PZT/ao1", "name to assign"="594 nm") -> ("task out"=w643:refnum<k21>)  [unwired: 10 in, 1 out]
          n252 = property class="DAQmx Timing"(reference=w567) -> ("SampClk.Rate"=w563:dbl)  [unwired: 1 in, 2 out]
          n253 = property class="DAQmx Channel"(reference=w568) -> ("CO.Pulse.Freq"=w566:dbl)  [unwired: 1 in, 2 out]
          n254 = property class="DAQmx Trigger"(reference=w606, error in=w522, "Start.Retriggerable"=w604) -> (reference out=w600:refnum<k21>, error out=w517:errorcluster)
          n255 = property class="DAQmx Trigger"(reference=w607, error in=w523, "Start.Retriggerable"=w604) -> (reference out=w601:refnum<k21>, error out=w518:errorcluster)
          n256 = property class="DAQmx Trigger"(reference=w605, error in=w521, "Start.Retriggerable"=w604) -> (reference out=w597:refnum<k21>, error out=w516:errorcluster)
          n257 = property class="DAQmx Trigger"(reference=w675, error in=w526, "Start.Retriggerable"=w604) -> (reference out=w674:refnum<k21>, error out=w515:errorcluster)
          n258 = property class="DAQmx Trigger"(reference=w684, error in=w525, "Start.Retriggerable"=w604) -> (reference out=w665:refnum<k21>, error out=w520:errorcluster)
          n259 = property class="DAQmx Trigger"(reference=w608, error in=w524, "Start.Retriggerable"=w604) -> (reference out=w609:refnum<k21>, error out=w519:errorcluster)
          n260 = property on="594 nm voltage" class="DigNum (strict)"() -> ("Value"=w644:dbl)  [unwired: 2 in, 2 out]
          n261 = property on="488  nm voltage" class="DigNum (strict)"() -> ("Value"=w634:dbl)  [unwired: 2 in, 2 out]
          n262 = case shown="False" w533 {
            tunnel: [0.99 w697] -> w534
            frame False {
            }
            frame True {
              n263 = property on="Pulse Duty Cycle" class="DigNum (strict)"() -> ("Value"=w699:dbl)  [unwired: 2 in, 2 out]
              n264 = Divide(x=w699, y=100.0) -> (x/y=w697:dbl)
            }
          }
          n265 = Multiply(x=w563, y=w561) -> (x*y=w529:dbl)
          n266 = call-poly <vilib>:"DAQmx Write.vi"("task/channels in"=w643, "data"=w644) -> ("task out"=w641:refnum<k21>, "error out"=w640:errorcluster)  [unwired: 11 in, 1 out]
          n267 = property class="DAQmx Timing"(reference=w600, error in=w517, "Sample Quantity:Sample Mode"=w508, "SampQuant.SampPerChan"=w529) -> (reference out=w599:refnum<k21>, error out=w510:errorcluster)
          n268 = property class="DAQmx Timing"(reference=w665, error in=w520, "Sample Quantity:Sample Mode"=w508, "SampQuant.SampPerChan"=w529) -> (reference out=w666:refnum<k21>, error out=w514:errorcluster)
          n269 = property class="DAQmx Timing"(reference=w601, error in=w518, "Sample Quantity:Sample Mode"=w508, "SampQuant.SampPerChan"=w593) -> (reference out=w602:refnum<k21>, error out=w511:errorcluster)
          n270 = property class="DAQmx Timing"(reference=w597, error in=w516, "Sample Quantity:Sample Mode"=w508, "SampQuant.SampPerChan"=w529) -> (reference out=w598:refnum<k21>, error out=w509:errorcluster)
          n271 = property class="DAQmx Timing"(reference=w609, error in=w519, "Sample Quantity:Sample Mode"=w508, "SampQuant.SampPerChan"=w592) -> (reference out=w603:refnum<k21>, error out=w512:errorcluster)
          n272 = Divide(x=1.0, y=w614) -> (x/y=w536:dbl)
          n273 = property class="DAQmx Timing"(reference=w641, error in=w640, "Sample Quantity:Sample Mode"=w642) -> (reference out=w639:refnum<k21>, error out=w638:errorcluster)
          n274 = call "make step function for duty cycle.vi"("amplitude"=w634, "period"=w536, "duty cycle"=w534, "sample rate"=w558) -> ("Waveform out"=w535:waveform(dbl))  [unwired: 7 in]
          n275 = call "galvo_triangle_wave.vi"("trial seconds"=w561, "final frequency"=w566, "amplitude"=w565, "sample rate"=w563) -> ("waveform array out"=w564:waveform(dbl)[])  [unwired: 7 in]
          n276 = call-poly <vilib>:"DAQmx Write.vi"("task/channels in"=w666, "data"=w564, "error in"=w514) -> ("task out"=w667:refnum<k21>, "error out"=w513:errorcluster)  [unwired: 10 in, 1 out]
          n277 = call <vilib>:"DAQmx Start Task.vi"("task/channels in"=w667, "error in"=w513) -> ("task out"=w571:refnum<k21>, "error out"=w501:errorcluster)  [unwired: 12 in]
          n278 = call <vilib>:"DAQmx Start Task.vi"("task/channels in"=w674, "error in"=w515) -> ("task out"=w673:refnum<k21>, "error out"=w502:errorcluster)  [unwired: 12 in]
          n279 = call <vilib>:"DAQmx Start Task.vi"("task/channels in"=w602, "error in"=w511) -> ("task out"=w590:refnum<k21>, "error out"=w497:errorcluster)  [unwired: 12 in]
          n280 = call <vilib>:"DAQmx Start Task.vi"("task/channels in"=w639, "error in"=w638) -> ("task out"=w582:refnum<k21>, "error out"=w505:errorcluster)  [unwired: 12 in]
          n281 = call <vilib>:"DAQmx Start Task.vi"("task/channels in"=w603, "error in"=w512) -> ("task out"=w584:refnum<k21>, "error out"=w498:errorcluster)  [unwired: 12 in]
          n282 = call-poly <vilib>:"DAQmx Write.vi"("task/channels in"=w549, "data"=w535, "error in"=w550) -> ("task out"=w559:refnum<k21>, "error out"=w556:errorcluster)  [unwired: 10 in, 1 out]
          n283 = call-poly <vilib>:"DAQmx Create Virtual Channel.vi"("initial count"=u32 0, "edge"=w671, "counter"=tag "GalvoPMT/ctr2") -> ("task out"=w683:refnum<k21>)  [unwired: 11 in, 1 out]
          n284 = property on="File prefix" class="Str"() -> ("Value"=w617:string)  [unwired: 2 in, 2 out]
          n285 = property class="DAQmx Channel"(reference=w683, "CI.CountEdges.Term"=w528, "CI.CountEdges.DigFltr.MinPulseWidth"=1e-06 ("DI.DigFltr.MinPulseWidth")) -> (reference out=w677:refnum<k21>)  [unwired: 1 in, 1 out]
          n286 = call-poly <vilib>:"DAQmx Trigger.vi"("task/channels in"=w559, "source"=w528, "error in"=w556) -> ("task out"=w554:refnum<k21>, "error out"=w555:errorcluster)  [unwired: 11 in]
          n287 = Concatenate Strings(w617, "_Kinetix.tdms") -> (w622:string)
          n288 = Concatenate Strings(w617, "_Zelux.tdms") -> (w618:string)
          n289 = String To Path(string=w618) -> (path=w619:path)
          n290 = String To Path(string=w622) -> (path=w620:path)
          n291 = property on="Save directory" class="Path"() -> ("Value"=w615:path)  [unwired: 2 in, 2 out]
          n292 = Build Path(base path=w615, name or relative path=w620) -> (appended path=w662:path)
          n293 = Build Path(base path=w615, name or relative path=w619) -> (appended path=w630:path)
          n294 = TDMS Open(10:T7."open or create" ("operation (0:open)"), 11:w630) -> (3:w532:refnum<k34>)  [unwired: 5 in, 1 out]
          n295 = TDMS Open(10:T7."open or create" ("operation (0:open)"), 11:w662) -> (3:w661:refnum<k34>)  [unwired: 5 in, 1 out]
          n296 = call <vilib>:"DAQmx Start Task.vi"("task/channels in"=w677) -> ("task out"=w676:refnum<k21>)  [unwired: 13 in, 1 out]
          n297 = call <vilib>:"DAQmx Start Task.vi"("task/channels in"=w554, "error in"=w555) -> ("task out"=w647:refnum<k21>, "error out"=w507:errorcluster)  [unwired: 12 in]
          n298 = while {
            tunnel: w611 -> [w719]
            tunnel: [w750] -> w681
            tunnel: [w749] -> w679
            tunnel: w676 -> [w746]
            tunnel: w673 -> [w724]
            tunnel: [FALSE] -> w591
            tunnel: w561 -> [w741]
            tunnel: w599 -> [w736]
            tunnel: [w738] -> w659
            tunnel: [w737] -> w658
            tunnel: [w735] -> w635
            tunnel: w647 -> [w735]
            tunnel: [w734] -> w633
            tunnel: [w733] -> w628
            tunnel: w598 -> [w732]
            tunnel: w590 -> [w727]
            tunnel: [w727] -> w587
            tunnel: w584 -> [w726]
            tunnel: [w726] -> w583
            tunnel: w582 -> [w725]
            tunnel: [w725] -> w575
            tunnel: [w724] -> w572
            tunnel: w571 -> [w723]
            tunnel: [w723] -> w570
            shift-right: [w721] -> w531
            shift-left: w532 -> [w722]
            shift-right: [w739] -> w660
            shift-left: w661 -> [w740]
            tunnel: w507 -> [w715]
            tunnel: [w715] -> w506
            tunnel: w505 -> [w714]
            tunnel: [w714] -> w504
            tunnel: w502 -> [w713]
            tunnel: [w713] -> w503
            tunnel: w501 -> [w712]
            tunnel: [w712] -> w500
            tunnel: w498 -> [w711]
            tunnel: [w711] -> w499
            tunnel: w497 -> [w710]
            tunnel: [w710] -> w496
            stop <- w745 stop-if-true
            # "Run experiment"
            n299 = Subtract(x=w719, y=u32 1 ("milliseconds to wait")) -> (x-y=w718:u32)
            n300 = call-poly <vilib>:"DAQmx Read.vi"("task/channels in"=w746) -> ("task out"=w750:refnum<k21>, "data"=w748:u32, "error out"=w749:errorcluster)  [unwired: 12 in]
            n301 = call-poly <vilib>:"DAQmx Read.vi"("task/channels in"=w732) -> ("task out"=w733:refnum<k21>, "data"=w709:waveform(dbl))  [unwired: 12 in, 1 out]
            n302 = call-poly <vilib>:"DAQmx Read.vi"("task/channels in"=w736) -> ("task out"=w737:refnum<k21>, "data"=w720:waveform(dbl))  [unwired: 12 in, 1 out]
            n303 = Wait (ms)(milliseconds to wait=u32 10) -> ()  [unwired: 1 out]
            n304 = Greater Or Equal?(x=w748, y=w718) -> (x >= y?=w743:bool)
            n305 = case shown="True" w743 {
              selector: w743 -> [w752 _]
              tunnel: [w752 w754] -> w742
              tunnel: w741 -> [_ w753]
              frame False {
              }
              frame True {
                n306 = while {
                  tunnel: [w755] -> w754
                  tunnel: w753 -> [w756]
                  stop <- w755 stop-if-true
                  n307 = call "Elapsed Time"("Time Target (s)"=w756) -> ("Time has Elapsed"=w755:bool)  [unwired: 11 in, 7 out]
                }
              }
            }
            n308 = call "extract TTL timing data.vi"("threshold"=1.0, "Waveform"=w709) -> ("x+y"=w729:timestamp[])  [unwired: 9 in]
            n309 = call "extract TTL timing data.vi"("threshold"=1.0, "Waveform"=w720) -> ("x+y"=w716:timestamp[])  [unwired: 9 in]
            n310 = TDMS Write(0:w740, 9:w716) -> (4:w739:refnum<k34>, 15:w738:errorcluster)  [unwired: 4 in, 2 out]
            n311 = TDMS Write(0:w722, 9:w729) -> (4:w721:refnum<k34>, 15:w734:errorcluster)  [unwired: 4 in, 2 out]
            n312 = Not(x="Begin Experiment") -> (.not. x?=w751:bool)
            n313 = Or(x=w742, y=w751) -> (x .or. y?=w745:bool)
          }
          n314 = call <vilib>:"DAQmx Stop Task.vi"("task/channels in"=w572, "error in"=w503) -> ("task out"=w574:refnum<k21>, "error out"=w573:errorcluster)  [unwired: 12 in]
          n315 = call <vilib>:"DAQmx Stop Task.vi"("task/channels in"=w681, "error in"=w679) -> ("task out"=w680:refnum<k21>, "error out"=w678:errorcluster)  [unwired: 12 in]
          n316 = call <vilib>:"DAQmx Stop Task.vi"("task/channels in"=w570, "error in"=w500) -> ("task out"=w541:refnum<k21>, "error out"=w539:errorcluster)  [unwired: 12 in]
          n317 = call <vilib>:"DAQmx Stop Task.vi"("task/channels in"=w587, "error in"=w496) -> ("task out"=w588:refnum<k21>, "error out"=w586:errorcluster)  [unwired: 12 in]
          n318 = property on="Begin Experiment" class="Bool (strict)"("Value"=w591) -> ()  [unwired: 2 in, 2 out]
          n319 = call <vilib>:"DAQmx Stop Task.vi"("task/channels in"=w583, "error in"=w499) -> ("task out"=w623:refnum<k21>, "error out"=w624:errorcluster)  [unwired: 12 in]
          n320 = call <vilib>:"DAQmx Clear Task.vi"("task in"=w574, "error in"=w573) -> ()  [unwired: 13 in, 1 out]
          n321 = call <vilib>:"DAQmx Clear Task.vi"("task in"=w680, "error in"=w678) -> ()  [unwired: 13 in, 1 out]
          n322 = call <vilib>:"DAQmx Stop Task.vi"("task/channels in"=w658, "error in"=w510) -> ("task out"=w664:refnum<k21>, "error out"=w663:errorcluster)  [unwired: 12 in]
          n323 = call <vilib>:"DAQmx Stop Task.vi"("task/channels in"=w628, "error in"=w509) -> ("task out"=w632:refnum<k21>, "error out"=w631:errorcluster)  [unwired: 12 in]
          n324 = call <vilib>:"DAQmx Stop Task.vi"("task/channels in"=w635, "error in"=w506) -> ("task out"=w636:refnum<k21>, "error out"=w637:errorcluster)  [unwired: 12 in]
          n325 = TDMS Close(8:w659, 11:w660) -> ()  [unwired: 2 out]
          n326 = TDMS Close(8:w633, 11:w531) -> ()  [unwired: 2 out]
          n327 = call <vilib>:"DAQmx Clear Task.vi"("task in"=w588, "error in"=w586) -> ("error out"=w585:errorcluster)  [unwired: 13 in]
          n328 = call <vilib>:"DAQmx Clear Task.vi"("task in"=w632, "error in"=w631) -> ()  [unwired: 13 in, 1 out]
          n329 = disable-structure shown="Disabled" {
            disable-tunnel: w637 -> [w693 w694]
            disable-tunnel: w636 -> [w692 w695]
            disable-tunnel: [w687 w695] -> w545
            disable-tunnel: [w686 w694] -> w542
            frame Disabled {
              n330 = Build Array(0.0) -> (w691:dbl[])
              n331 = Bundle By Name("Y"=w691) -> (w689:waveform(dbl))  [unwired: 1 in]
              n332 = call-poly <vilib>:"DAQmx Write.vi"("task/channels in"=w692, "auto start"=TRUE, "data"=w689, "error in"=w693) -> ("task out"=w687:refnum<k21>, "error out"=w686:errorcluster)  [unwired: 9 in, 1 out]
            }
            frame Enabled {
            }
          }
          n333 = call <vilib>:"DAQmx Clear Task.vi"("task in"=w664, "error in"=w663) -> ()  [unwired: 13 in, 1 out]
          n334 = call <vilib>:"DAQmx Clear Task.vi"("task in"=w623, "error in"=w624) -> ("error out"=w626:errorcluster)  [unwired: 13 in]
          n335 = property class="DAQmx Timing"(reference=w541, "Sample Quantity:Sample Mode"=w538) -> (reference out=w540:refnum<k21>)  [unwired: 1 in, 1 out]
          n336 = call <vilib>:"DAQmx Stop Task.vi"("task/channels in"=w575, "error in"=w504) -> ("task out"=w578:refnum<k21>, "error out"=w579:errorcluster)  [unwired: 12 in]
          n337 = call <vilib>:"Simple Error Handler.vi"("type of dialog (OK msg:1)"=w625, "error in (no error)"=w626) -> ()  [unwired: 3 in, 5 out]
          n338 = call <vilib>:"Simple Error Handler.vi"("type of dialog (OK msg:1)"=w589, "error in (no error)"=w585) -> ()  [unwired: 3 in, 5 out]
          n339 = disable-structure shown="Enabled" {
            disable-tunnel: w579 -> [w705 w707]
            disable-tunnel: w578 -> [w704 w708]
            disable-tunnel: [w701 w708] -> w577
            disable-tunnel: [w700 w707] -> w576
            frame Disabled {
              n340 = call-poly <vilib>:"DAQmx Write.vi"("task/channels in"=w704, "data"=0.0, "error in"=w705) -> ("task out"=w703:refnum<k21>, "error out"=w702:errorcluster)  [unwired: 10 in, 1 out]
              n341 = call <vilib>:"DAQmx Start Task.vi"("task/channels in"=w703, "error in"=w702) -> ("task out"=w701:refnum<k21>, "error out"=w700:errorcluster)  [unwired: 12 in]
            }
            frame Enabled {
            }
          }
          n342 = call "galvo_recenter.vi"("error in"=w539, "task/channels in"=w540) -> ()  [unwired: 10 in]
          n343 = call <vilib>:"DAQmx Wait Until Done.vi"("task/channels in"=w545, "error in"=w542) -> ("task out"=w544:refnum<k21>, "error out"=w543:errorcluster)  [unwired: 12 in]
          n344 = call <vilib>:"DAQmx Clear Task.vi"("task in"=w577, "error in"=w576) -> ("error out"=w581:errorcluster)  [unwired: 13 in]
          n345 = call <vilib>:"Simple Error Handler.vi"("type of dialog (OK msg:1)"=w580, "error in (no error)"=w581) -> ()  [unwired: 3 in, 5 out]
          n346 = call <vilib>:"DAQmx Clear Task.vi"("task in"=w544, "error in"=w543) -> ("error out"=w646:errorcluster)  [unwired: 13 in]
          n347 = call <vilib>:"Simple Error Handler.vi"("type of dialog (OK msg:1)"=w645, "error in (no error)"=w646) -> ()  [unwired: 3 in, 5 out]
        }
      }
    }
    frame Disabled {
    }
  }
  n348 = property on="Run Live" class="Bool (strict)"("Caption.Text"=w33) -> ()  [unwired: 2 in, 2 out]
  n349 = case shown="True" w30 {
    tunnel: "scan/fast camera frequency" -> [_ w764]
    tunnel: "Galvo voltage" -> [_ w804]
    tunnel: "slow camera frequency" -> [_ w763]
    tunnel: "Pulse Duty Cycle" -> [_ w788]
    frame False {
    }
    frame True {
      w769 = T8 0 items=["no dialog", "OK message", "continue or stop message", "OK message + warnings", "continue/stop + warnings"] ("type of dialog (OK msg:1)")
      w778 = 0.0
      w795 = T8 0 items=["no dialog", "OK message", "continue or stop message", "OK message + warnings", "continue/stop + warnings"] ("type of dialog (OK msg:1)")
      w819 = T8 0 items=["no dialog", "OK message", "continue or stop message", "OK message + warnings", "continue/stop + warnings"] ("type of dialog (OK msg:1)")
      w821 = T8 0 items=["no dialog", "OK message", "continue or stop message", "OK message + warnings", "continue/stop + warnings"] ("type of dialog (OK msg:1)")
      # "run galvo/camera trigger \n(and shutter trigger) continuously"
      n350 = call "init_DAQ_cluster.vi"("Slow/Zelux frame frequency"=w763, "Fast/Kinetix frame frequency"=w764) -> ("error out"=w757:errorcluster, "tasks cluster"=w762:T9)  [unwired: 8 in]
      n351 = Unbundle By Name(w762) -> ("shutter trigger"=w760:refnum<k21>, "galvo control"=w758:refnum<k21>, "Kinetix trigger"=w759:refnum<k21>, "Zelux trigger"=w761:refnum<k21>)
      n352 = property class="DAQmx Channel"(reference=w759, error in=w757) -> ("CO.Pulse.Freq"=w803:dbl)  [unwired: 2 out]
      n353 = property class="DAQmx Timing"(reference=w758) -> ("SampClk.Rate"=w802:dbl)  [unwired: 1 in, 2 out]
      n354 = property on="594 nm voltage" class="DigNum (strict)"() -> ("Value"=w783:dbl)  [unwired: 2 in, 2 out]
      n355 = call <vilib>:"DAQmx Start Task.vi"("task/channels in"=w760, "error in"=w757) -> ("task out"=w818:refnum<k21>, "error out"=w816:errorcluster)  [unwired: 12 in]
      n356 = call "galvo_triangle_wave.vi"("final frequency"=w803, "amplitude"=w804, "sample rate"=w802) -> ("waveform array out"=w810:waveform(dbl)[])  [unwired: 8 in]
      n357 = property on="488  nm voltage" class="DigNum (strict)"() -> ("Value"=w784:dbl)  [unwired: 2 in, 2 out]
      n358 = Divide(x=w788, y=100.0) -> (x/y=w787:dbl)
      n359 = call-poly <vilib>:"DAQmx Write.vi"("task/channels in"=w758, "data"=w810, "error in"=w757) -> ("task out"=w830:refnum<k21>, "error out"=w829:errorcluster)  [unwired: 10 in, 1 out]
      n360 = Bundle By Name(cluster=T10 {"voltage"=0.0, "frequency"=0.0, "duty cycle"=0.0, "sample rate"=1000.0} ("channel parameters"), "voltage"=w784, "frequency"=w763, "duty cycle"=w787, "sample rate"=10000.0) -> (w782:T10)
      n361 = call <vilib>:"DAQmx Start Task.vi"("task/channels in"=w761, "error in"=w757) -> ("task out"=w772:refnum<k21>, "error out"=w771:errorcluster)  [unwired: 12 in]
      n362 = call <vilib>:"DAQmx Start Task.vi"("task/channels in"=w759, "error in"=w757) -> ("task out"=w824:refnum<k21>, "error out"=w823:errorcluster)  [unwired: 12 in]
      n363 = property on="Pulse 488" class="Bool (strict)"() -> ("Value"=w790:bool)  [unwired: 2 in, 2 out]
      n364 = call "init_lasers.vi"("488 pulsed"=w790, "594 nm voltage"=w783, "488 nm channel parameters"=w782) -> ("error out"=w800:errorcluster, "task out"=w801:refnum<k21>)  [unwired: 6 in, 1 out]
      n365 = call <vilib>:"DAQmx Start Task.vi"("task/channels in"=w830, "error in"=w829) -> ("task out"=w825:refnum<k21>, "error out"=w826:errorcluster)  [unwired: 12 in]
      n366 = property on="Run time" class="DigNum (strict)"() -> ("Value"=w806:i32)  [unwired: 2 in, 2 out]
      n367 = Equal To 0?(x=w806) -> (x = 0?=w807:bool)
      n368 = while {
        tunnel: w825 -> [w856]
        tunnel: w826 -> [w855]
        tunnel: [w845] -> w828
        tunnel: [w854] -> w827
        tunnel: w824 -> [w852]
        tunnel: w823 -> [w847]
        tunnel: [w847] -> w814
        tunnel: [w852] -> w812
        tunnel: w818 -> [w849]
        tunnel: [w849] -> w817
        tunnel: w816 -> [w846]
        tunnel: [w846] -> w815
        tunnel: w807 -> [w841]
        tunnel: w806 -> [w840]
        tunnel: [FALSE] -> w805
        tunnel: w801 -> [w838]
        tunnel: w800 -> [w837]
        tunnel: [w836] -> w799
        tunnel: [w835] -> w798
        tunnel: w782 -> [w833]
        tunnel: [w831] -> w766
        tunnel: w772 -> [w831]
        tunnel: [w832] -> w765
        tunnel: w771 -> [w832]
        stop <- w839 stop-if-true
        n369 = event shown="[0] Timeout" {
          selector: _ -> [_ _ _]
          dyn-events: _ -> [_ _ _]
          timeout: 50 -> [_ _ _]
          tunnel: w837 -> [w863 w908 w911]
          tunnel: [w857 w907 w910] -> w836
          tunnel: [w862 w908 w911] -> w835
          tunnel: w838 -> [w861 w907 w910]
          tunnel: w833 -> [w860 _ _]
          event Timeout {
            n370 = flat-sequence {
              tunnel: w863 -> [w871]
              tunnel: w861 -> [w869]
              tunnel: w860 -> [w864]
              tunnel: [w870] -> w859
              tunnel: [w865] -> w858
              tunnel: [w905] -> w857
              tunnel: [w906] -> w862
              tunnel: w859 -> [w906]
              tunnel: w858 -> [w905]
              frame #0 {
                n371 = property on="594 changed" class="Bool (strict)"() -> ("Value"=w866:bool)  [unwired: 2 in, 2 out]
                n372 = property on="488 changed" class="Bool (strict)"() -> ("Value"=w867:bool)  [unwired: 2 in, 2 out]
                n373 = Or(x=w867, y=w866) -> (x .or. y?=w868:bool)
                n374 = case shown="True" w868 {
                  tunnel: w871 -> [w873 w884]
                  tunnel: [w872 w883] -> w865
                  tunnel: [w873 w882] -> w870
                  tunnel: w869 -> [w872 w879]
                  tunnel: w864 -> [_ w876]
                  frame False {
                  }
                  frame True {
                    n375 = local read "488 nm LED control"() -> (w875:dbl)
                    n376 = local read "594 nm laser control"() -> (w874:dbl)
                    n377 = Divide(x=w875, y=20.0) -> (x/y=w881:dbl)
                    n378 = Divide(x=w874, y=20.0) -> (x/y=w880:dbl)
                    n379 = property on="Pulse 488" class="Bool (strict)"() -> ("Value"=w885:bool)  [unwired: 2 in, 2 out]
                    n380 = case shown="True" w885 {
                      tunnel: [w893 w900] -> w882
                      tunnel: w884 -> [w892 w901]
                      tunnel: w879 -> [w890 w902]
                      tunnel: [w891 w903] -> w883
                      tunnel: w881 -> [w888 w896]
                      tunnel: w880 -> [w887 w898]
                      tunnel: w876 -> [_ w895]
                      frame False {
                        n381 = Build Array(w888, w887) -> (w886:dbl[])
                        n382 = call-poly <vilib>:"DAQmx Write.vi"("task/channels in"=w890, "auto start"=TRUE, "data"=w886, "error in"=w892) -> ("task out"=w891:refnum<k21>, "error out"=w893:errorcluster)  [unwired: 9 in, 1 out]
                      }
                      frame True {
                        n383 = Bundle By Name(cluster=w895, "voltage"=w896) -> (w894:T10)
                        n384 = call "pulse 488 and steady 594.vi"("594 amplitude"=w898, "488 nm channel parameters"=w894) -> ("waveforms out"=w897:waveform(dbl)[])  [unwired: 9 in]
                        n385 = call-poly <vilib>:"DAQmx Write.vi"("task/channels in"=w902, "auto start"=TRUE, "data"=w897, "error in"=w901) -> ("task out"=w903:refnum<k21>, "error out"=w900:errorcluster)  [unwired: 9 in, 1 out]
                      }
                    }
                  }
                }
              }
              frame #1 {
                w904 = FALSE ("488 changed")
                n386 = property on="488 changed" class="Bool (strict)"("Value"=w904) -> ()  [unwired: 2 in, 2 out]
                n387 = property on="594 changed" class="Bool (strict)"("Value"=w904) -> ()  [unwired: 2 in, 2 out]
              }
            }
            n388 = event-data() -> ()  [unwired: 1 in, 1 out]
          }
          event "488 nm LED control": Mouse Up {
            n389 = event-data() -> ()  [unwired: 1 in, 8 out]
            "488 changed" <- TRUE ("488 changed")
          }
          event "594 nm laser control": Mouse Up {
            n390 = event-data() -> ()  [unwired: 1 in, 8 out]
            "594 changed" <- TRUE
          }
        }
        n391 = call <vilib>:"DAQmx Is Task Done.vi"("task/channels in"=w856, "error in"=w855) -> ("task out"=w854:refnum<k21>, "error out"=w845:errorcluster)  [unwired: 11 in, 1 out]
        n392 = Merge Errors(w847, w846, w845) -> (w848:errorcluster)
        n393 = case shown="False" w841 {
          tunnel: [w914 FALSE] -> w843
          tunnel: w840 -> [w913 _]
          frame False {
            n394 = call "Elapsed Time2"("Time Target (s)"=w913) -> ("Time has Elapsed"=w914:bool)  [unwired: 11 in, 7 out]
          }
          frame True {
          }
        }
        n395 = Unbundle By Name(w848) -> ("status"=w853:bool)
        n396 = Not(x="Run Live") -> (.not. x?=w851:bool)
        n397 = Or(x=w853, y=w851) -> (x .or. y?=w844:bool)
        n398 = Or(x=w844, y=w843) -> (x .or. y?=w839:bool)
      }
      n399 = property on="Run Live" class="Bool (strict)"("Value"=w805) -> ()  [unwired: 2 in, 2 out]
      n400 = property on="594 nm laser control" class="Slide (strict)"() -> ("Value"=w777:dbl)  [unwired: 2 in, 2 out]
      n401 = call <vilib>:"DAQmx Clear Task.vi"("task in"=w817, "error in"=w815) -> ("error out"=w820:errorcluster)  [unwired: 13 in]
      n402 = call <vilib>:"DAQmx Stop Task.vi"("task/channels in"=w766, "error in"=w765) -> ("task out"=w767:refnum<k21>, "error out"=w768:errorcluster)  [unwired: 12 in]
      n403 = call <vilib>:"DAQmx Stop Task.vi"("task/channels in"=w827, "error in"=w828) -> ("task out"=w809:refnum<k21>, "error out"=w808:errorcluster)  [unwired: 12 in]
      n404 = call <vilib>:"DAQmx Stop Task.vi"("task/channels in"=w812, "error in"=w814) -> ("task out"=w811:refnum<k21>, "error out"=w813:errorcluster)  [unwired: 12 in]
      n405 = call <vilib>:"DAQmx Stop Task.vi"("task/channels in"=w799, "error in"=w798) -> ("task out"=w796:refnum<k21>, "error out"=w797:errorcluster)  [unwired: 12 in]
      n406 = Divide(x=w777, y=20.0) -> (x/y=w775:dbl)
      n407 = call "galvo_recenter.vi"("error in"=w808, "task/channels in"=w809) -> ()  [unwired: 10 in]
      n408 = Build Array(w778, w778, w778, w778) -> (w780:dbl[])
      n409 = call <vilib>:"Simple Error Handler.vi"("type of dialog (OK msg:1)"=w819, "error in (no error)"=w820) -> ()  [unwired: 3 in, 5 out]
      n410 = Build Array(w775, w775, w775, w775) -> (w774:dbl[])
      n411 = call <vilib>:"DAQmx Clear Task.vi"("task in"=w767, "error in"=w768) -> ("error out"=w770:errorcluster)  [unwired: 13 in]
      n412 = call <vilib>:"DAQmx Clear Task.vi"("task in"=w811, "error in"=w813) -> ("error out"=w822:errorcluster)  [unwired: 13 in]
      n413 = Bundle By Name("Y"=w780) -> (w781:waveform(dbl))  [unwired: 1 in]
      n414 = Bundle By Name("Y"=w774) -> (w773:waveform(dbl))  [unwired: 1 in]
      n415 = call <vilib>:"Simple Error Handler.vi"("type of dialog (OK msg:1)"=w769, "error in (no error)"=w770) -> ()  [unwired: 3 in, 5 out]
      n416 = call <vilib>:"Simple Error Handler.vi"("type of dialog (OK msg:1)"=w821, "error in (no error)"=w822) -> ()  [unwired: 3 in, 5 out]
      n417 = Build Array(w781, w773) -> (w779:waveform(dbl)[])
      n418 = call-poly <vilib>:"DAQmx Write.vi"("task/channels in"=w796, "auto start"=TRUE, "data"=w779, "error in"=w797) -> ("task out"=w793:refnum<k21>, "error out"=w792:errorcluster)  [unwired: 9 in, 1 out]
      n419 = call <vilib>:"DAQmx Clear Task.vi"("task in"=w793, "error in"=w792) -> ("error out"=w794:errorcluster)  [unwired: 13 in]
      n420 = call <vilib>:"Simple Error Handler.vi"("type of dialog (OK msg:1)"=w795, "error in (no error)"=w794) -> ()  [unwired: 3 in, 5 out]
    }
  }
  n421 = event shown="[0] Timeout" {
    selector: _ -> [_ _ _]
    dyn-events: _ -> [_ _ _]
    timeout: 2 -> [_ _ _]
    event Timeout {
      n422 = event-data() -> ()  [unwired: 1 in, 3 out]
    }
    event "Connect Zelux": Value Change {
      n423 = event-data() -> ("NewVal"=w916:bool)  [unwired: 1 in, 5 out]
      n424 = case shown="True" w916 {
        frame False {
        }
        frame True {
        }
      }
    }
    event "Connect Kinetix": Value Change {
      n425 = event-data() -> ("NewVal"=w917:bool)  [unwired: 1 in, 5 out]
      n426 = case shown="False" w917 {
        frame False {
          # "shut down camera"
          n427 = property on="Camera obj" class="LVClassControl (strict)"() -> ("Value"=w919:refnum<class "Camera.lvclass">)  [unwired: 2 in, 2 out]
          n428 = property on="PVCam error out" class="Clust (strict)"() -> ("Value"=w921:errorcluster)  [unwired: 2 in, 2 out]
          n429 = call "Close Camera.vi"("error in (no error)"=w921, "Camera in"=w919) -> ("error out"=w918:errorcluster)  [unwired: 8 in, 1 out]
          n430 = property on="PVCAM Out" class="LVClassControl (strict)"() -> ("Value"=w920:refnum<class "PVCAM.lvclass">)  [unwired: 2 in, 2 out]
          n431 = call "Release.vi"("error in (no error)"=w918, "PVCAM in"=w920) -> ()  [unwired: 8 in, 2 out]
        }
        frame True {
          n432 = call "PV_setup.vi"() -> ("error out"=→"PVCam error out":errorcluster, "Camera out"=→"Camera obj":refnum<class "Camera.lvclass">, "PVCAM Out"=→"PVCAM Out":refnum<class "PVCAM.lvclass">)  [unwired: 7 in, 2 out]
        }
      }
    }
  }
  n433 = disable-structure shown="Enabled" {
    frame Disabled {
      n434 = Open VI Reference(vi path=path "C:/Users/Thor/Documents/MM_LabView/laser_LED_controls.vi") -> (vi reference=w925:refnum<vi>, error out=w926:errorcluster)  [unwired: 5 in]
    }
    frame Enabled {
    }
  }
  n435 = property on="Begin Experiment" class="Bool (strict)"("Caption.Text"=w25) -> ()  [unwired: 2 in, 2 out]
  n436 = disable-structure shown="Enabled" {
    frame Disabled {
      w941 = T8 0 items=["no dialog", "OK message", "continue or stop message", "OK message + warnings", "continue/stop + warnings"] ("type of dialog (OK msg:1)")
      (unwired) 0.0 ("voltage")
      (unwired) 0.0 ("frequency")
      (unwired) 0.0 ("duty cycle")
      (unwired) 0.0 ("sample rate")
      n437 = property on="Property Node" class="DigNum (strict)"() -> ("Value"=w951:dbl)  [unwired: 2 in, 2 out]
      n438 = property on="Property Node" class="DigNum (strict)"() -> ("Value"=w952:dbl)  [unwired: 2 in, 2 out]
      n439 = Bundle By Name("voltage"=w952, "duty cycle"=w951) -> (w949:cluster{}, w943:cluster{}, "sample rate"=w950:dbl)  [unwired: 1 in]
      n440 = disable-structure shown="Disabled" {
        disable-tunnel: [w982 w991] -> w945
        disable-tunnel: [w981 w990] -> w944
        disable-tunnel: w943 -> [w980 _]
        frame Disabled {
          n441 = property on="Property Node" class="DigNum (strict)"() -> ("Value"=w984:dbl)  [unwired: 2 in, 2 out]
          n442 = Bundle By Name(cluster=w980, "voltage"=w984, "sample rate"=1000.0) -> (w986:cluster{})
          n443 = call "init_laser.vi"("Pulsed"=FALSE, "Voltage limits"=T11 {"maximum value"=5.0, "minimum value"=0.0}, "channel parameters"=w986, "name to assign"="594 nm", "physical channels"=tag "PZT/ao1") -> ("error out"=w981:errorcluster, "task out"=w982:refnum<k21>)  [unwired: 5 in]
        }
        frame Enabled {
          n444 = disable-structure shown="Enabled" {
            disable-tunnel: [w993 w996] -> w991
            disable-tunnel: [errorcluster {"status"=FALSE, "code"=0, "source"=""} ("error constant") w995] -> w990
            frame Disabled {
              w993 = refnum<k21> refnum  # DAQmx Task Name
            }
            frame Enabled {
              n445 = call-poly <vilib>:"DAQmx Create Virtual Channel.vi"("physical channels"=tag "PZT/ao1") -> ("task out"=w996:refnum<k21>, "error out"=w995:errorcluster)  [unwired: 13 in]
            }
          }
        }
      }
      n446 = property on="Property Node" class="Bool (strict)"() -> ("Value"=w946:bool)  [unwired: 2 in, 2 out]
      n447 = call "init_laser.vi"("Pulsed"=w946, "Voltage limits"=T11 {"maximum value"=5.0, "minimum value"=0.0}, "channel parameters"=w949, "name to assign"="488 nm", "physical channels"=tag "PZT/ao0") -> ("error out"=w947:errorcluster, "task out"=w948:refnum<k21>)  [unwired: 5 in]
      n448 = event shown="[1] Timeout" {
        selector: _ -> [_ _ _]
        dyn-events: _ -> [_ _ _]
        timeout: 0 -> [_ _ _]
        tunnel: [w963 w966 w974] -> w936
        tunnel: [w962 w967 w973] -> w935
        tunnel: [w961 w966 w974] -> w929
        tunnel: [w960 w967 w973] -> w930
        tunnel: [w959 w968 w971] -> w934
        tunnel: [w959 w968 w975] -> w933
        tunnel: [w958 w969 w976] -> w932
        tunnel: [w958 w969 w972] -> w931
        event #0 (no event record) {
          n449 = event-data() -> ("NewVal"=w957)  [unwired: 1 in, 5 out]
          n450 = Divide(x=w957, y=20.0) -> (x/y=w964:dbl)
          n451 = call-poly <vilib>:"DAQmx Write.vi"("task/channels in"=w963, "auto start"=TRUE, "data"=w964, "error in"=w962) -> ("task out"=w961:refnum<k21>, "error out"=w960:errorcluster)  [unwired: 9 in, 1 out]
        }
        event Timeout {
          n452 = event-data() -> ()  [unwired: 1 in, 3 out]
        }
        event #2 (no event record) {
          n453 = event-data() -> ("NewVal"=w978)  [unwired: 1 in, 5 out]
          n454 = Divide(x=w978, y=20.0) -> (x/y=w977:dbl)
          n455 = call-poly <vilib>:"DAQmx Write.vi"("task/channels in"=w972, "auto start"=TRUE, "data"=w977, "error in"=w971) -> ("task out"=w976:refnum<k21>, "error out"=w975:errorcluster)  [unwired: 9 in, 1 out]
        }
      }
      n456 = call <vilib>:"DAQmx Clear Task.vi"() -> ("error out"=w942:errorcluster)  [unwired: 15 in]
      n457 = call <vilib>:"DAQmx Stop Task.vi"() -> ("task/channels in"=w939:refnum<k21>, "task out"=w938:refnum<k21>, "error in"=w940:errorcluster, "error out"=w937:errorcluster)  [unwired: 12 in]
      n458 = call <vilib>:"Simple Error Handler.vi"("type of dialog (OK msg:1)"=w941, "error in (no error)"=w942) -> ()  [unwired: 3 in, 5 out]
      n459 = call "clear_laser.vi"("error in"=w937, "task/channels in"=w938) -> ()  [unwired: 10 in]
    }
    frame Enabled {
    }
  }
